vi "BRig_RT_panel_Laser2_v1,13.vi"(7 "input_setValues":bool, 9 "input_dataExp":u16[](array[numeric]), 11 "input_dataLC":u16[](array[numeric])) -> (1 "output_dataExp":u16[](array[numeric]), 3 "output_dataLC":u16[](array[numeric]))   [LabVIEW 2014]
panel:
  in  "LC_Wro_nRew2":u16
  in  "LC_Wro_nRew1":u16
  in  "LC_Rew_nRew2":u16
  in  "LC_Rew_nRew1":u16
  in  "LC_Sel_nRew2":u16
  in  "LC_Sel_nRew1":u16
  in  "LC_Cue2_nRew2":u16
  in  "LC_Cue2_nRew1":u16
  in  "LC_Cue_nRew2":u16
  in  "LC_Cue_nRew1":u16
  in  "LC_ENL2_nRew2":u16
  in  "LC_ENL2_nRew1":u16
  in  "LC_ENL_nRew2":u16
  in  "LC_ENL_nRew1":u16
  in  "LC_Cue2_PostR_Count":u16
  in  "LC_Cue2_PostR_delayOpt":bool
  in  "LC_Cue2_PostR_Probability":u16
  in  "LC_Cue2_PostR_Block":u16(slide) max=2 step=1 scale=0.0..2.0
  in  "LC_Cue2_PostR_OnOff":bool
  in  "LC_Cue2_PostR_Tdelay":u16
  in  "LC_ENL2_PostR_delayOpt":bool
  in  "LC_ENL2_PostR_Count":u16
  in  "LC_ENL2_PostR_Probability":u16 max=100 step=1
  in  "LC_ENL2_PostR_Block":u16(slide) max=2 step=1 scale=0.0..2.0
  in  "LC_ENL2_PostR_OnOff":bool
  in  "LC_ENL2_PostR_Tdelay":u16
  in  "LC_Cue2_PreR_Count":u16
  in  "LC_Cue2_First_Count":u16
  in  "LC_Cue2_PreR_delayOpt":bool
  in  "LC_ENL2_PreR_delayOpt":bool
  in  "LC_ENL2_PreR_Count":u16
  in  "LC_ENL2_First_Count":u16
  in  "LC_Cue2_First_delayOpt":bool
  in  "LC_ENL2_First_delayOpt":bool
  in  "LC_Cue2_PreR_Probability":u16
  in  "LC_Cue2_PreR_Block":u16(slide) max=2 step=1 scale=0.0..2.0
  in  "LC_Cue2_PreR_OnOff":bool
  in  "LC_Cue2_First_Probability":u16
  in  "LC_Cue2_First_Block":u16(slide) max=2 step=1 scale=0.0..2.0
  in  "LC_Cue2_First_OnOff":bool
  in  "LC_ENL2_PreR_Probability":u16 max=100 step=1
  in  "LC_ENL2_PreR_Block":u16(slide) max=2 step=1 scale=0.0..2.0
  in  "LC_ENL2_PreR_OnOff":bool
  in  "LC_ENL2_First_Probability":u16 max=100 step=1
  in  "LC_ENL2_First_Block":u16(slide) max=2 step=1 scale=0.0..2.0
  in  "LC_Cue2_PreR_Tdelay":u16
  in  "LC_ENL2_PreR_Tdelay":u16
  in  "LC_Cue2_First_Tdelay":u16
  in  "LC_ENL2_First_Tdelay":u16
  in  "LC_ENL2_First_OnOff":bool
  out "LaserPulseTrain":cluster{u16[], u16[]}(graph)
  in  "LED_baseline":bool
  in  "Laser_power_step":dbl
  in  "Laser_power_max":dbl
  in  "Laser_power_min":dbl
  in  "Laser_Tshutter":u16=2
  in  "Laser_Freq":u16=10
  in  "Laser_Tpeak":u16=2
  in  "Laser_T":u16
  in  "LC_Sel_PostR_Count":u16
  in  "LC_Sel_PostR_Probability":u16
  in  "LC_Sel_PostR_Block":u16(slide) max=2 step=1 scale=0.0..2.0
  in  "LC_Sel_PostR_OnOff":bool
  in  "LC_Sel_PostR_Tdelay":u16
  in  "LC_Cue_PostR_Count":u16
  in  "LC_Cue_PostR_delayOpt":bool
  in  "LC_Cue_PostR_Probability":u16
  in  "LC_Cue_PostR_Block":u16(slide) max=2 step=1 scale=0.0..2.0
  in  "LC_Cue_PostR_OnOff":bool
  in  "LC_Cue_PostR_Tdelay":u16
  in  "LC_ENL_PostR_delayOpt":bool
  in  "LC_ENL_PostR_Count":u16
  in  "LC_ENL_PostR_Probability":u16 max=100 step=1
  in  "LC_ENL_PostR_Block":u16(slide) max=2 step=1 scale=0.0..2.0
  in  "LC_ENL_PostR_OnOff":bool
  in  "LC_ENL_PostR_Tdelay":u16
  in  "LC_Sel_PreR_Count":u16
  in  "LC_Sel_First_Count":u16
  in  "LC_Sel_PreR_Probability":u16
  in  "LC_Sel_PreR_Block":u16(slide) max=2 step=1 scale=0.0..2.0
  in  "LC_Sel_PreR_OnOff":bool
  in  "LC_Sel_First_Probability":u16
  in  "LC_Sel_First_Block":u16(slide) max=2 step=1 scale=0.0..2.0
  in  "LC_Sel_First_OnOff":bool
  in  "LC_Sel_PreR_Tdelay":u16
  in  "LC_Sel_First_Tdelay":u16
  in  "LC_Cue_PreR_Count":u16
  in  "LC_Cue_First_Count":u16
  in  "LC_Cue_PreR_delayOpt":bool
  in  "LC_ENL_PreR_delayOpt":bool
  in  "LC_ENL_PreR_Count":u16
  in  "LC_ENL_First_Count":u16
  in  "LC_Cue_First_delayOpt":bool
  in  "LC_ENL_First_delayOpt":bool
  in  "LC_Wrong_Probability":u16
  in  "LC_Wrong_Trial":u16(slide) max=4 step=1 scale=0.0..4.0
  in  "LC_Wrong_Block":u16(slide) max=2 step=1 scale=0.0..2.0
  in  "LC_Wrong_OnOff":bool
  in  "LC_Reward_Probability":u16
  in  "LC_Reward_Trial":u16(slide) max=3 step=1 scale=0.0..3.0
  in  "LC_Reward_Block":u16(slide) max=2 step=1 scale=0.0..2.0
  in  "LC_Reward_OnOff":bool
  in  "LC_Cue_PreR_Probability":u16
  in  "LC_Cue_PreR_Block":u16(slide) max=2 step=1 scale=0.0..2.0
  in  "LC_Cue_PreR_OnOff":bool
  in  "LC_Cue_First_Probability":u16
  in  "LC_Cue_First_Block":u16(slide) max=2 step=1 scale=0.0..2.0
  in  "LC_Cue_First_OnOff":bool
  in  "LC_ENL_PreR_Probability":u16 max=100 step=1
  in  "LC_ENL_PreR_Block":u16(slide) max=2 step=1 scale=0.0..2.0
  in  "LC_ENL_PreR_OnOff":bool
  in  "LC_ENL_First_Probability":u16 max=100 step=1
  in  "LC_ENL_First_Block":u16(slide) max=2 step=1 scale=0.0..2.0
  in  "LC_Wrong_Tdelay":u16
  in  "LC_Cue_PreR_Tdelay":u16
  in  "LC_ENL_PreR_Tdelay":u16
  in  "LC_Reward_Tdelay":u16
  in  "LC_Cue_First_Tdelay":u16
  in  "LC_ENL_First_Tdelay":u16
  in  "LC_ENL_First_OnOff":bool
  # "Laser2 Control\n                               On/Off      Block        Probability [%]   Delay [ms]                              Count"
  # "On/Off      Block        Probability [%]   Delay [ms]                              Count"
  # "Enforced\nNonLick"
  # "Enforced\nNonLick\n     2"
  # "from end"
  # "from end"
  # "First\nTrial"
  # "First\nTrial"
  # "from start"
  # "from start"
  # "from end"
  # "from end"
  # "PreReward\nTrials"
  # "PreReward\nTrials"
  # "from start"
  # "from start"
  # "from end"
  # "from end"
  # "PostReward\nTrials"
  # "PostReward\nTrials"
  # "from start"
  # "from start"
  # "PostReward Option - Trigger after [X1] or [X2] reward\n                                        (0 = ignore this option)"
  # "PostReward Option - Trigger after [X1] or [X2] reward\n                                        (0 = ignore this option)"
  # "Cue"
  # "Cue\n  2"
  # "from end"
  # "from end"
  # "First\nTrial"
  # "First\nTrial"
  # "from start"
  # "from start"
  # "from end"
  # "from end"
  # "PreReward\nTrials"
  # "PreReward\nTrials"
  # "from start"
  # "from start"
  # "from end"
  # "from end"
  # "PostReward\nTrials"
  # "PostReward\nTrials"
  # "from start"
  # "from start"
  # "PostReward Option - Trigger after [X1] or [X2] reward\n                                        (0 = ignore this option)"
  # "PostReward Option - Trigger after [X1] or [X2] reward\n                                        (0 = ignore this option)"
  # "Selection"
  # "from start"
  # "First\nTrial"
  # "from start"
  # "PreReward\nTrials"
  # "from start"
  # "PostReward\nTrials"
  # "PostReward Option - Trigger after [X1] or [X2] reward\n                                        (0 = ignore this option)"
  # "Laser2 Parameters"
  # "Laser2 Response\n           On/Off      Block           Trial     Probability %  Delay [ms]"
  # "Frequency\n[Hz]"
  # "Selection\nReward"
  # "Timing [ms]\n Duration     Peak Width   Shutter"
  # "Trigger after [X1] or [X2] reward\n(0 = ignore this option)"
  # "Laser Power [V]\nMin          Max              Step"
  # "Selection\nWrong"
  # "Trigger after [X1] or [X2] reward\n(0 = ignore this option)"
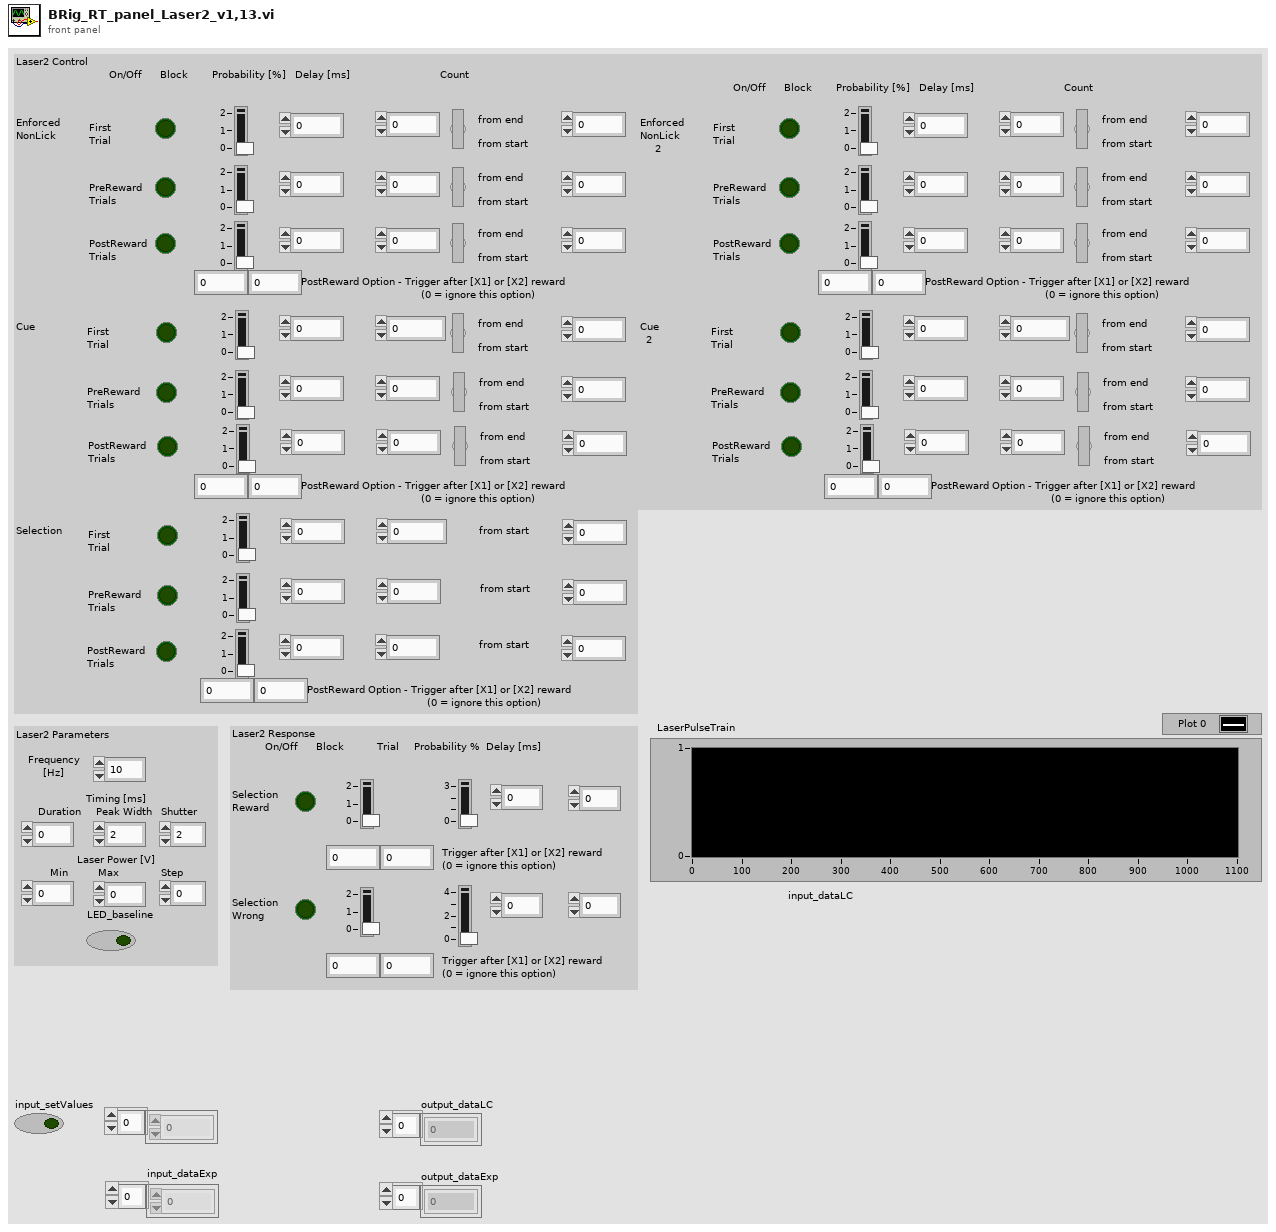
[diagram p1: front panel]
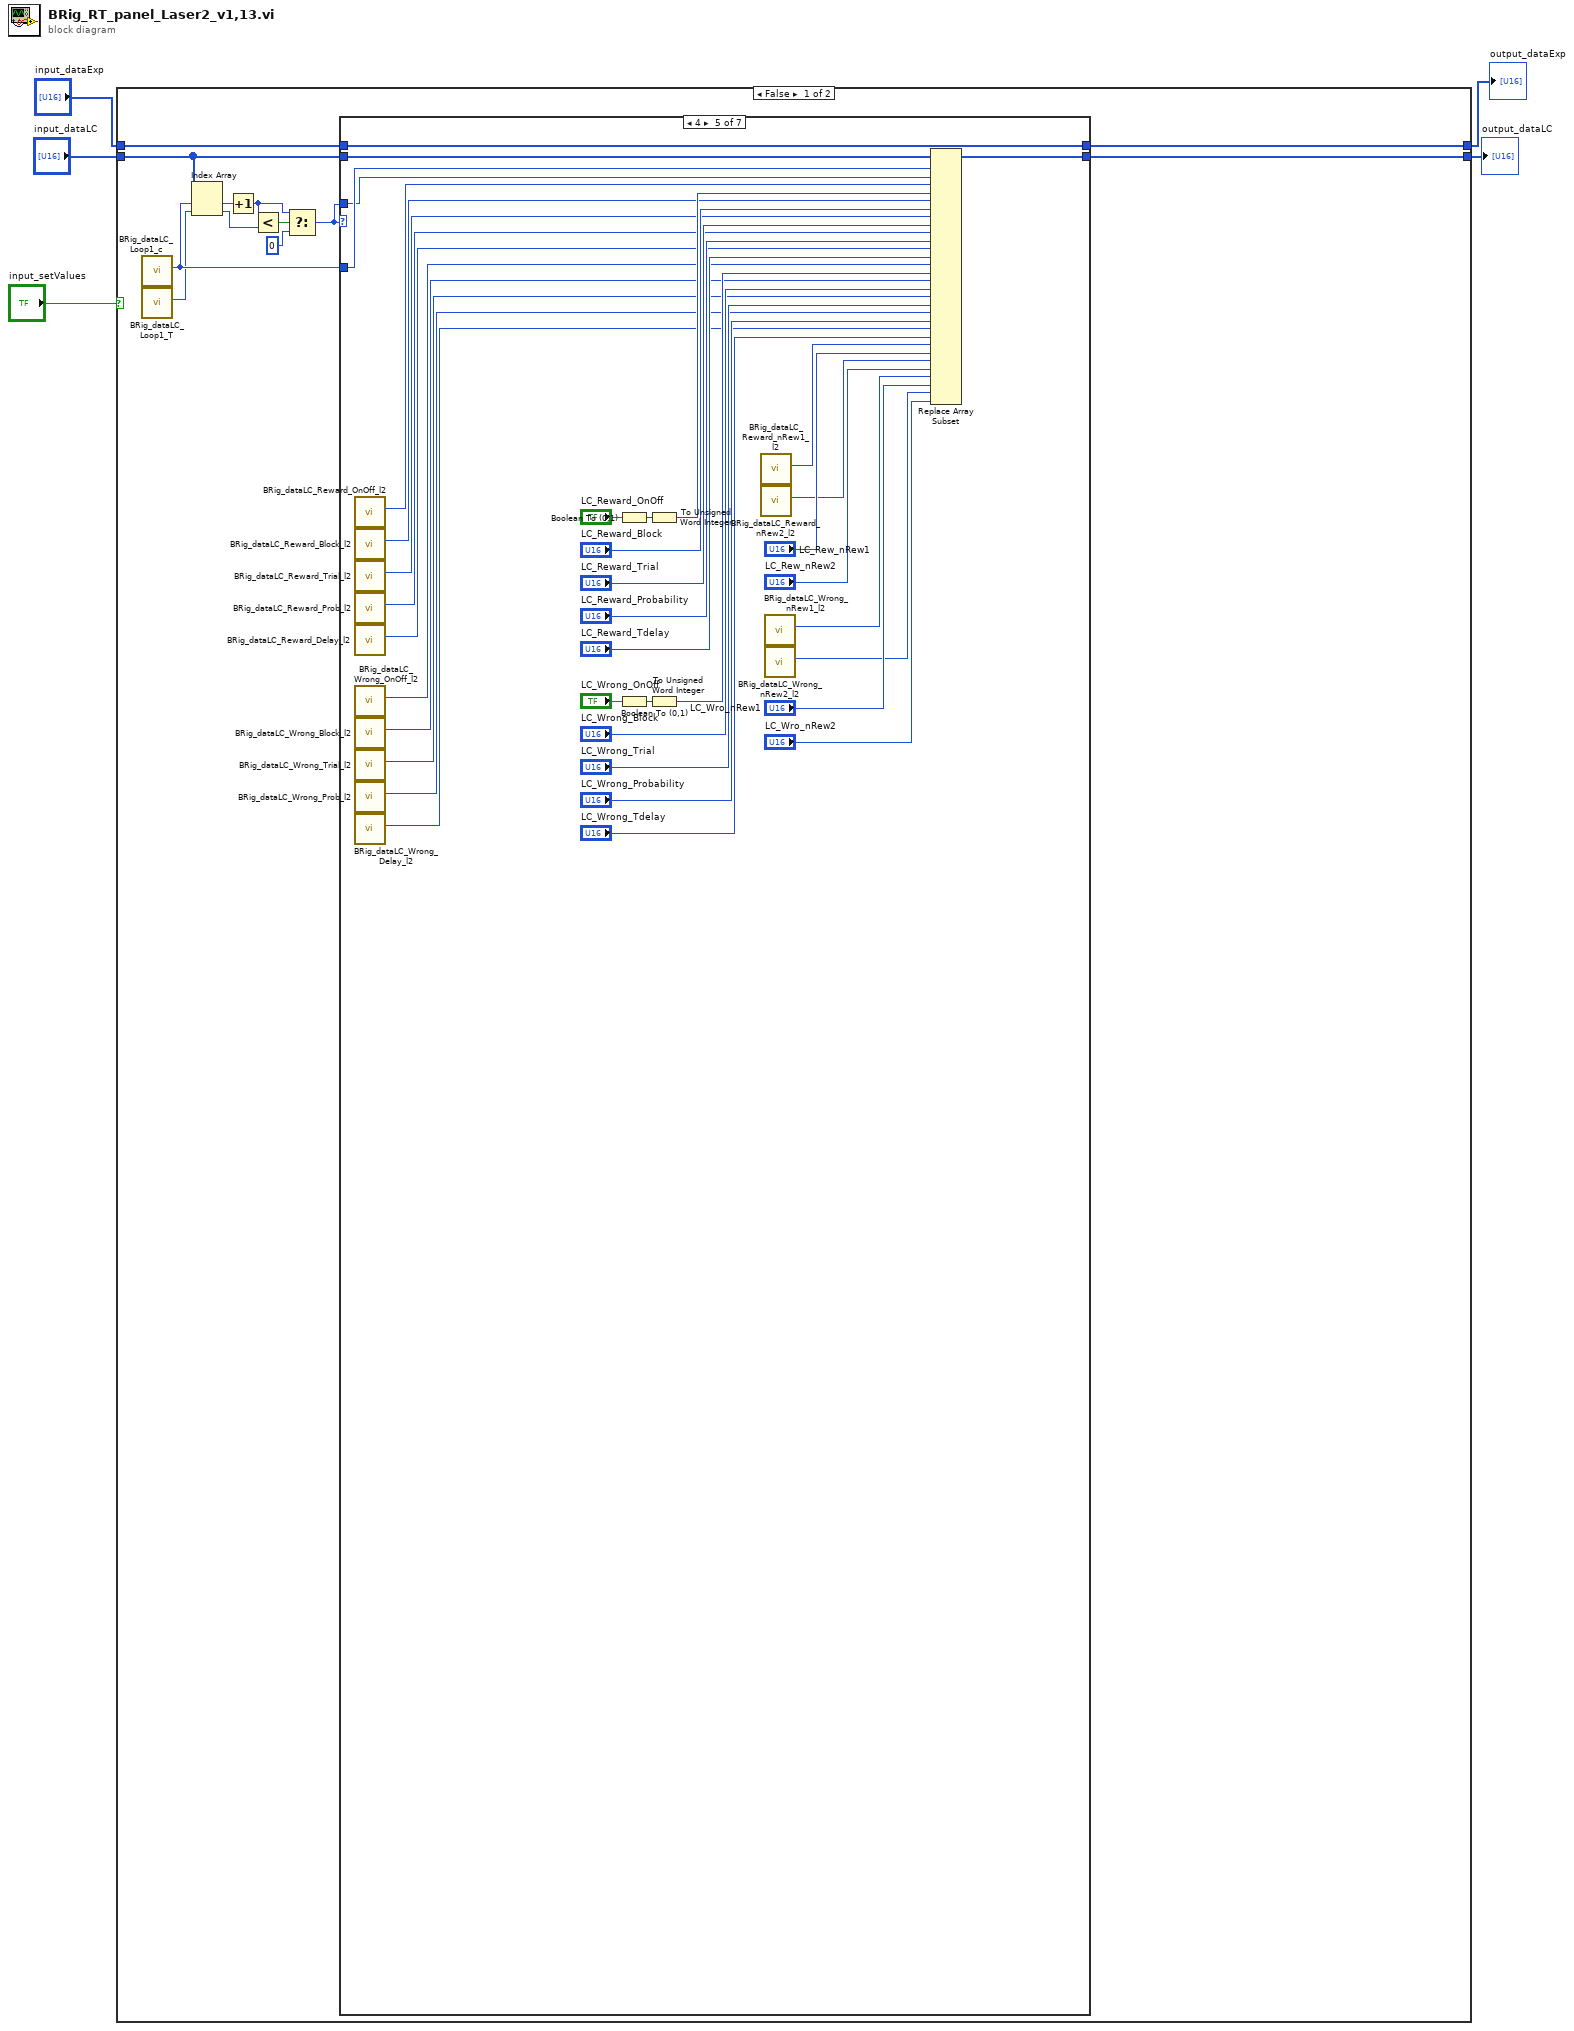
[diagram p0: block diagram]
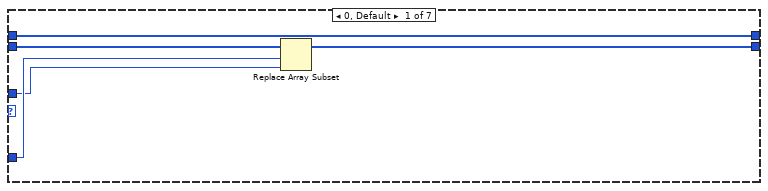
[diagram p2: hidden frame]
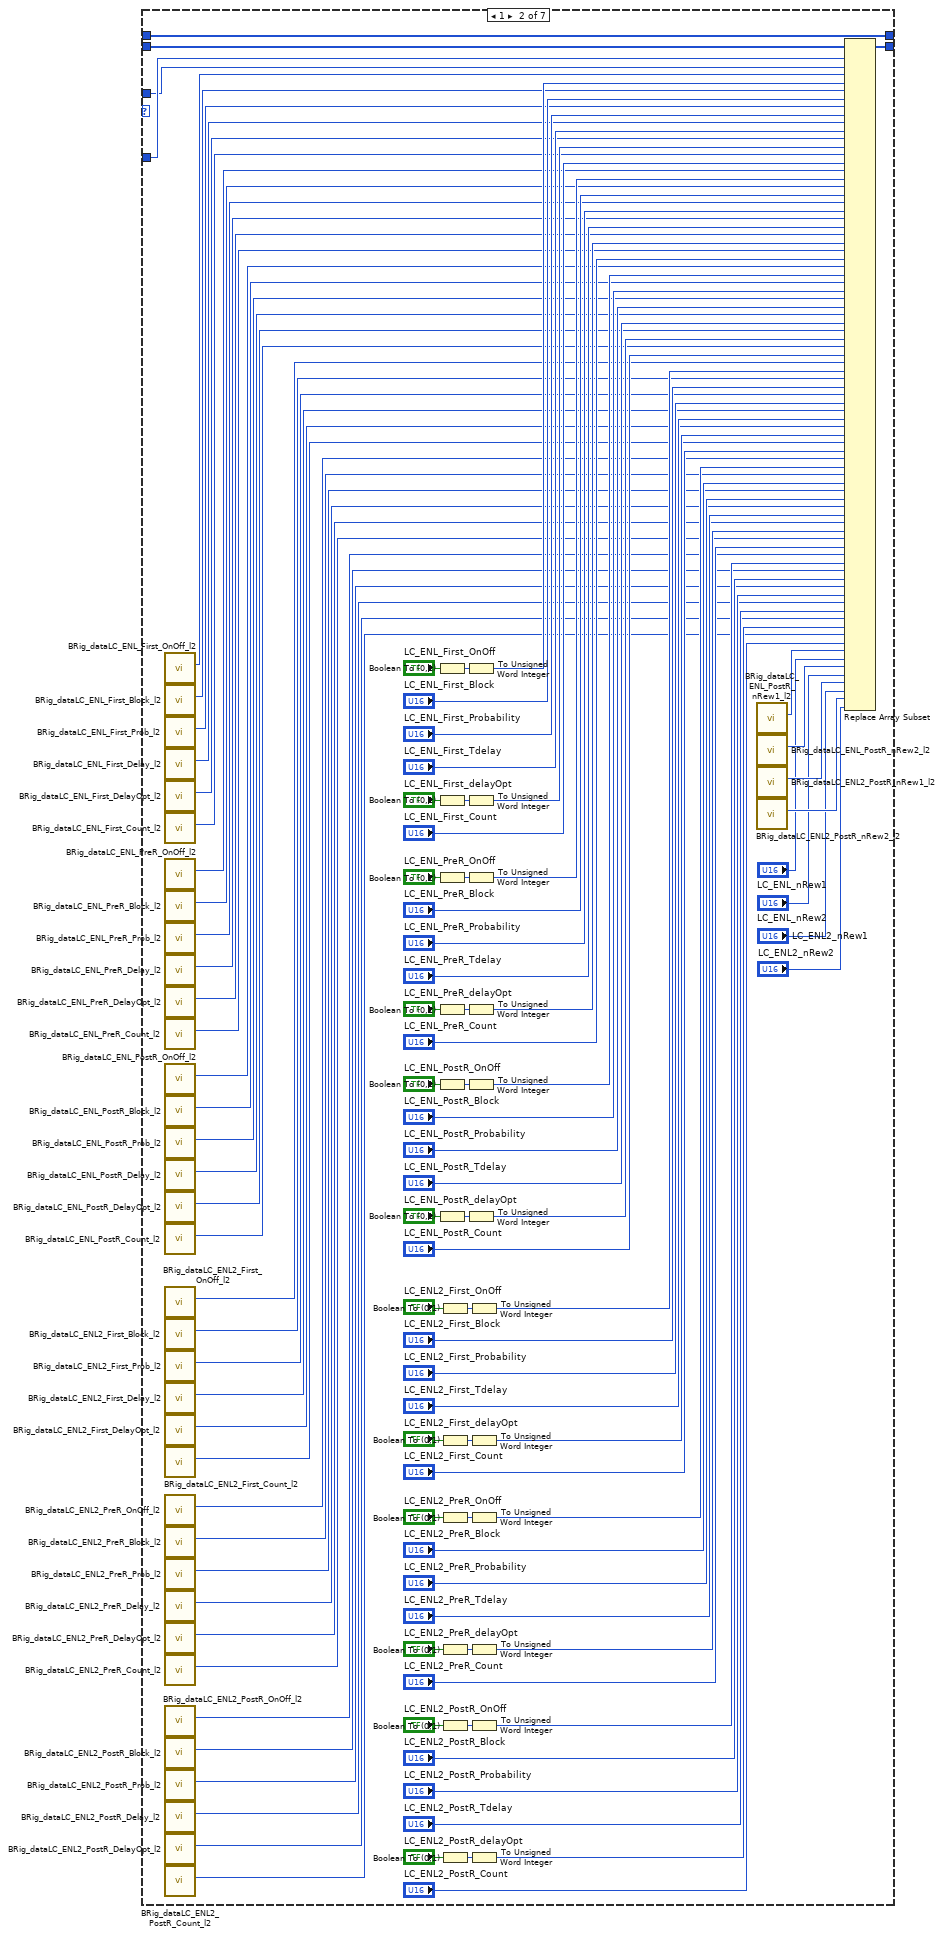
[diagram p3: hidden frame]
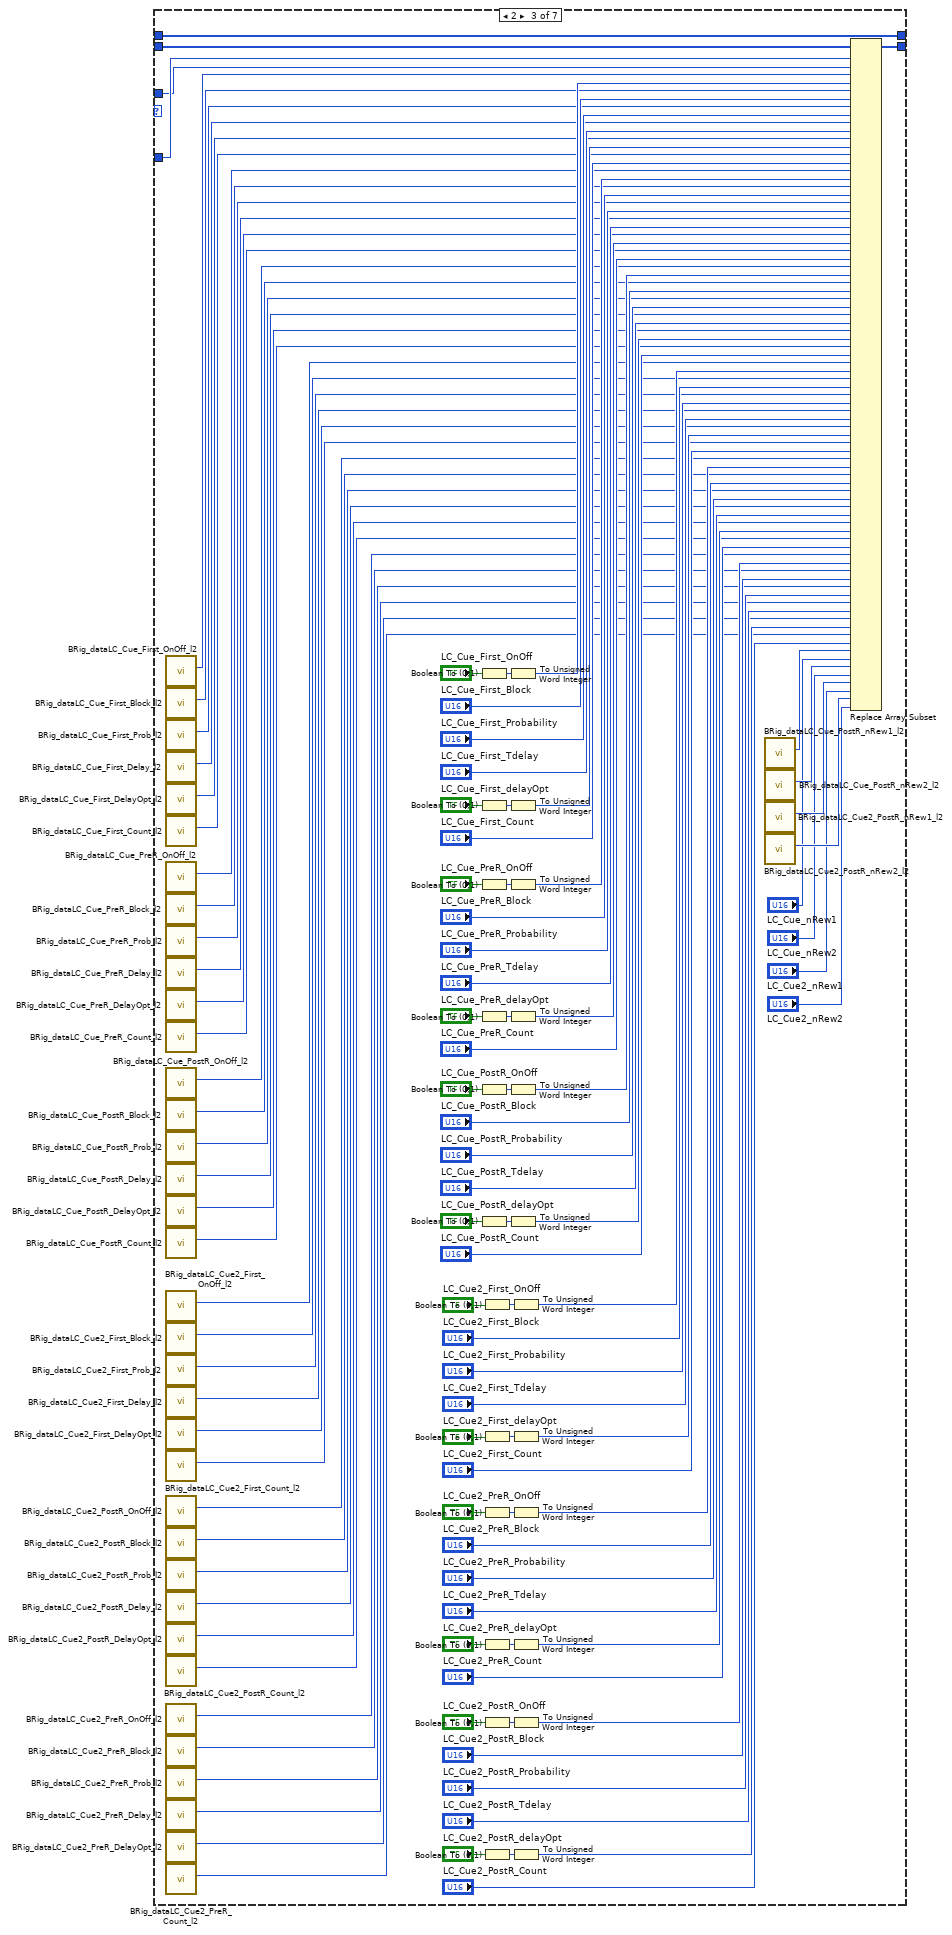
[diagram p4: hidden frame]
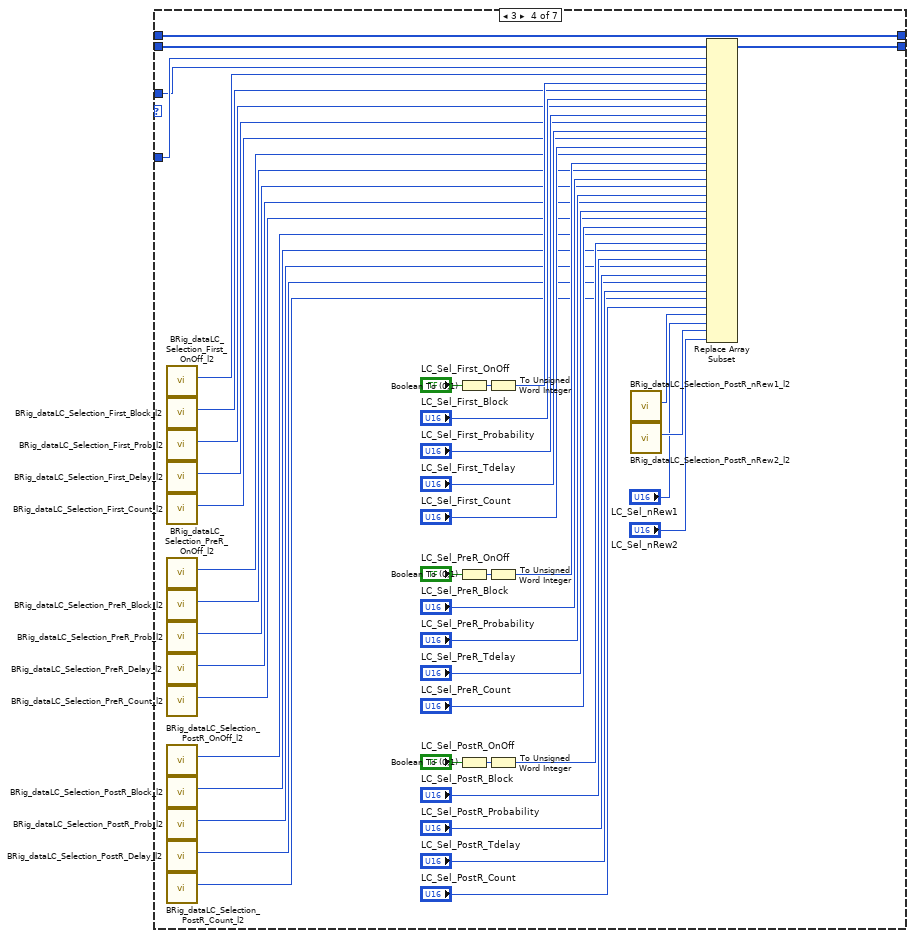
[diagram p5: hidden frame]
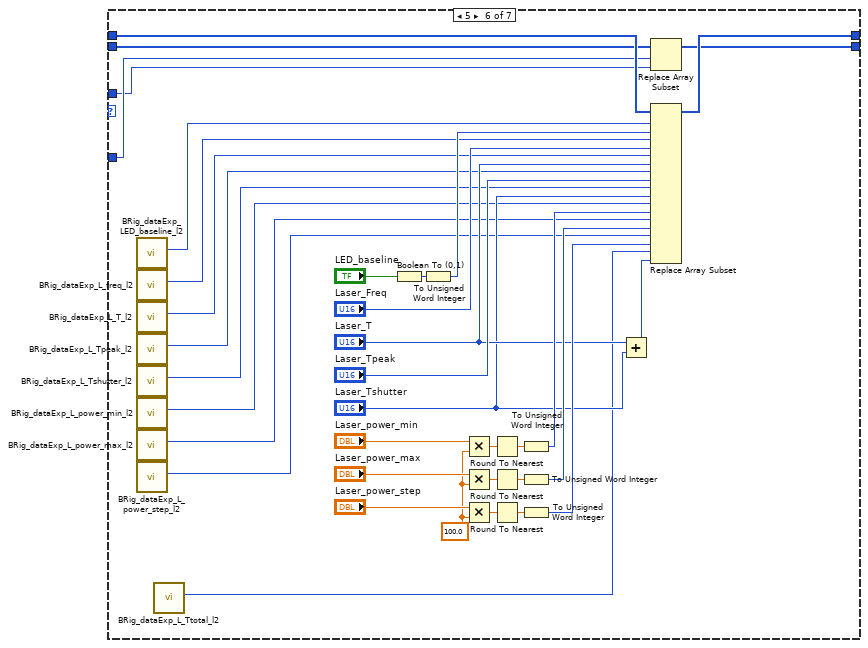
[diagram p6: hidden frame]
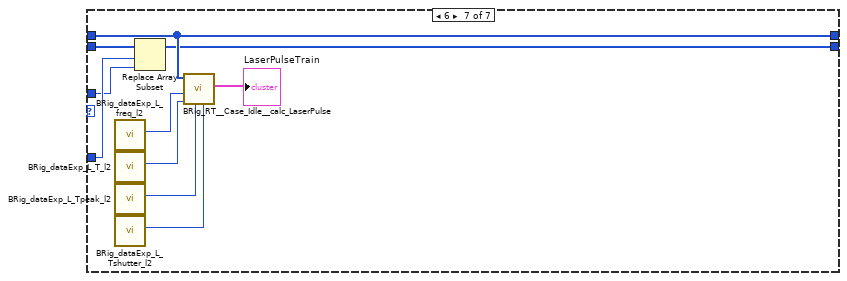
[diagram p7: hidden frame]
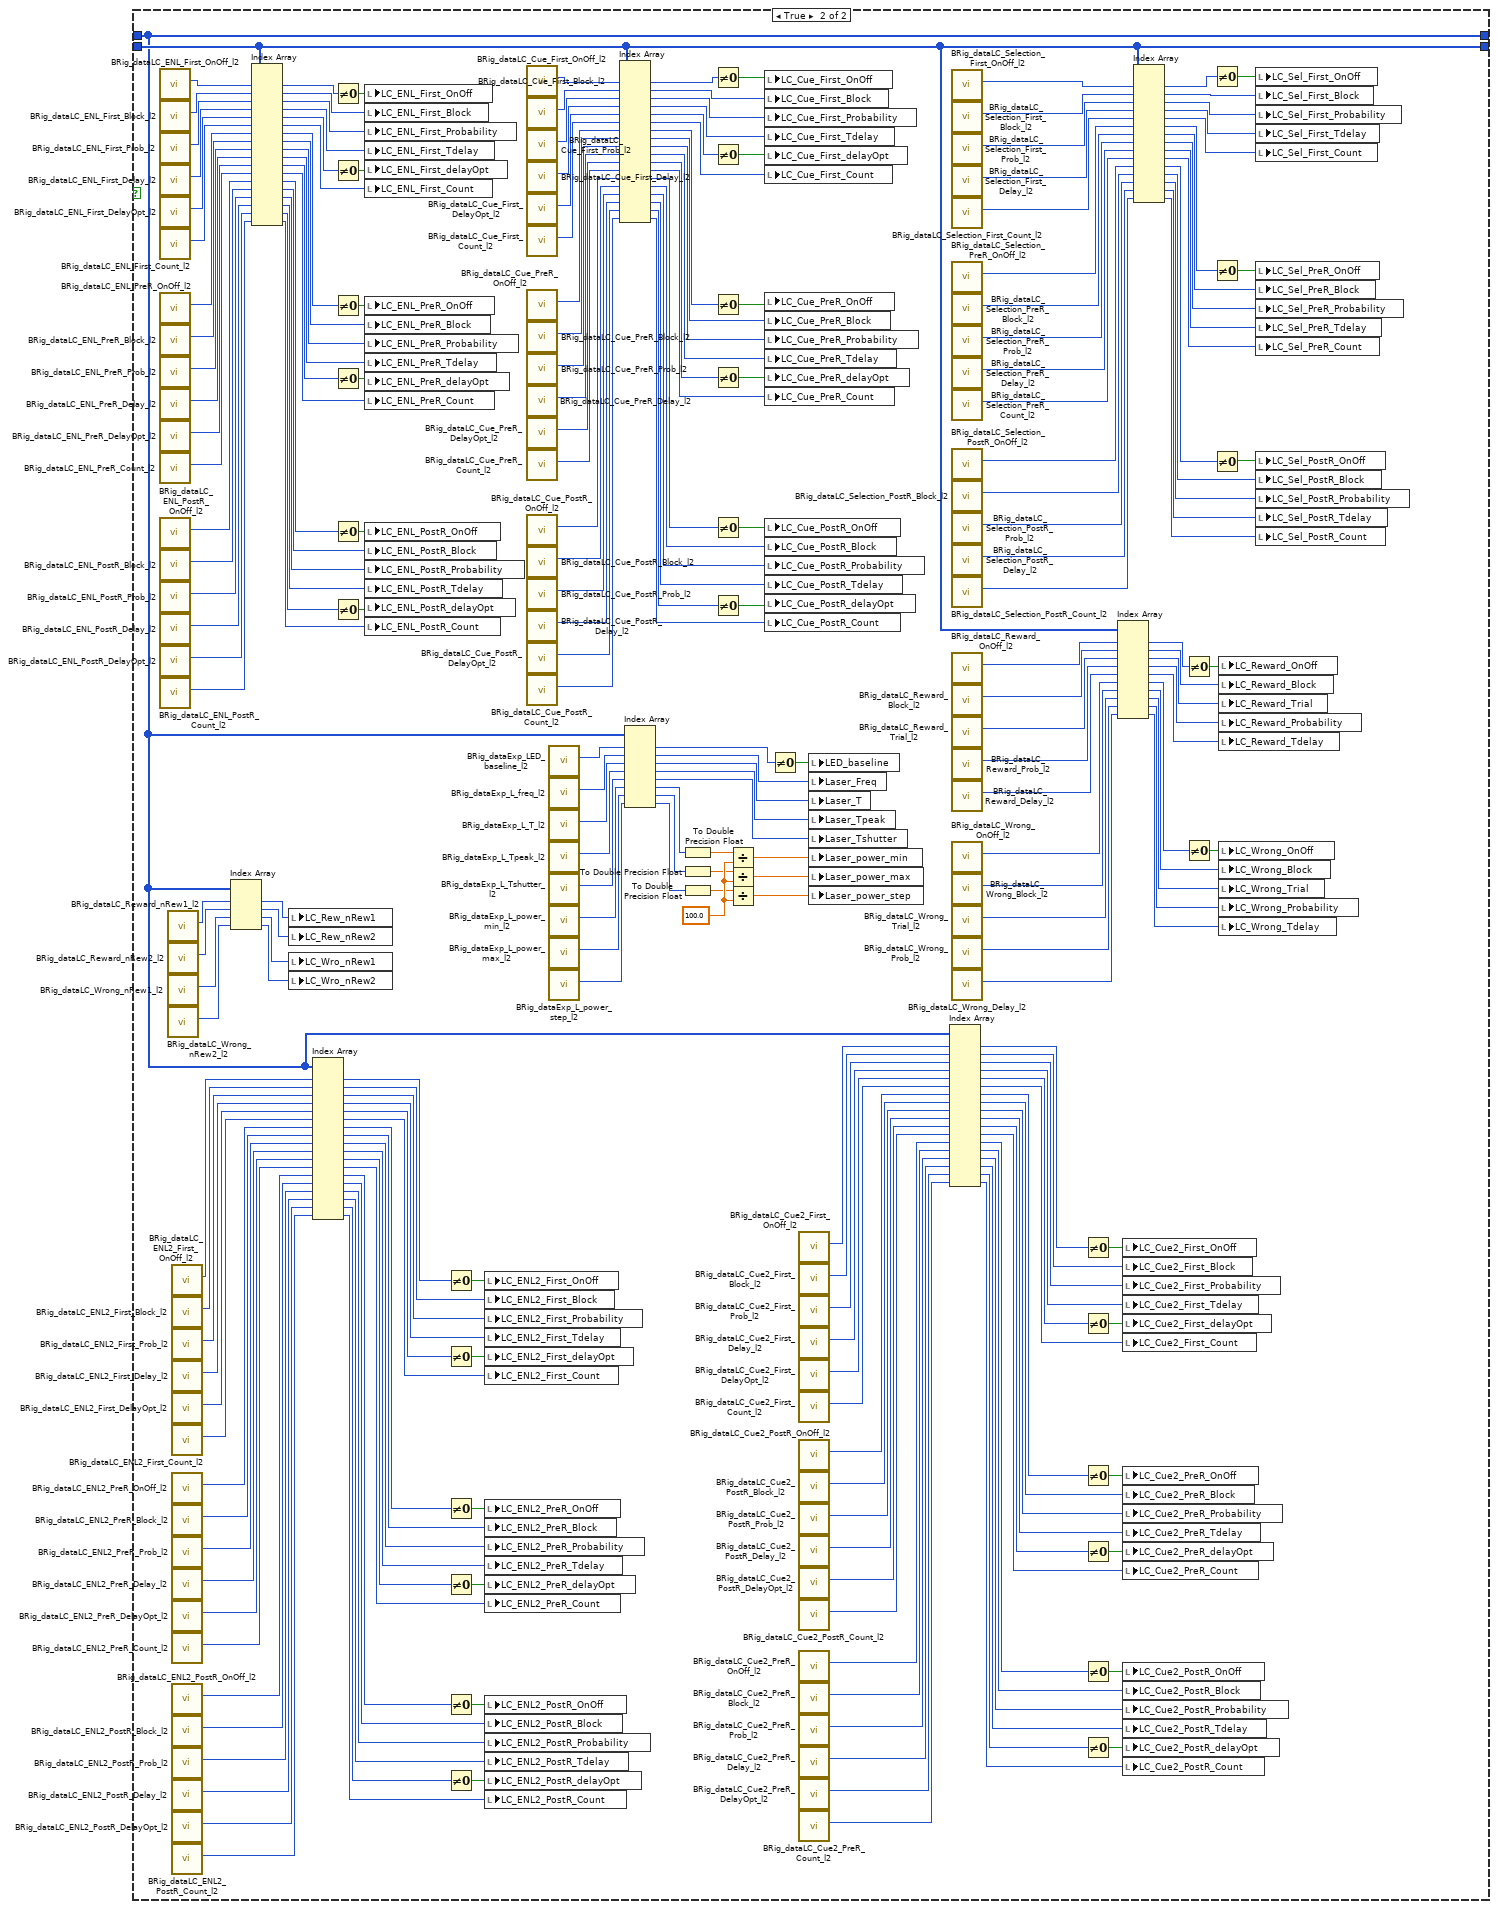
[diagram p8: hidden frame]
diagram:
  n1 = case shown="False" "input_setValues" {
    tunnel: "input_dataLC" -> [w17 w547]
    tunnel: [w11 w547] -> w4
    tunnel: "input_dataExp" -> [w7 w377]
    tunnel: [w6 w377] -> w1
    frame False {
      n2 = call "BRig_dataLC_Loop1_c.vi"() -> ("output_Loop1_c"=w10:i32)  [unwired: 11 in]
      n3 = call "BRig_dataLC_Loop1_T.vi"() -> ("output_Loop1_T"=w9:i32)  [unwired: 11 in]
      n4 = Index Array(array=w17, index #1=w10, index #2=w9) -> (element #1=w16:u16, element #2=w15:u16)
      n5 = Increment(x=w16) -> (x+1=w12:u16)
      n6 = Less?(x=w12, y=w15) -> (x < y?=w14:bool)
      n7 = Select(t=w12, s=w14, f=u16 0) -> (s? t:f=w8:u16)
      n8 = case shown="4" w8 {
        tunnel: w17 -> [w22 w131 w240 w285 w322 w335 w366]
        tunnel: w10 -> [w20 w99 w208 w262 w306 w333 w364]
        tunnel: w8 -> [w19 w98 w207 w261 w305 w332 w363]
        tunnel: [w21 w130 w239 w284 w321 w334 w365] -> w11
        tunnel: w7 -> [w18 w97 w206 w260 w304 w337 w368]
        tunnel: [w18 w97 w206 w260 w304 w336 w368] -> w6
        frame 0, Default {
          n9 = Replace Array Subset(array=w22, new element=w19, index=w20) -> (w21:u16[])
        }
        frame 1 {
          n10 = call "BRig_dataLC_ENL_First_OnOff_l2.vi"() -> ("output_ENL_First_OnOff_l2"=w49:i32)  [unwired: 11 in]
          n11 = call "BRig_dataLC_ENL_First_Block_l2.vi"() -> ("output_ENL_First_Block_l2"=w50:i32)  [unwired: 11 in]
          n12 = call "BRig_dataLC_ENL_First_Prob_l2.vi"() -> ("output_ENL_First_Prob_l2"=w51:i32)  [unwired: 11 in]
          n13 = call "BRig_dataLC_ENL_First_Delay_l2.vi"() -> ("output_ENL_First_Delay_l2"=w52:i32)  [unwired: 11 in]
          n14 = call "BRig_dataLC_ENL_First_DelayOpt_l2.vi"() -> ("output_ENL_First_DelayOpt_l2"=w53:i32)  [unwired: 11 in]
          n15 = call "BRig_dataLC_ENL_First_Count_l2.vi"() -> ("output_ENL_First_Count_l2"=w54:i32)  [unwired: 11 in]
          n16 = call "BRig_dataLC_ENL_PreR_OnOff_l2.vi"() -> ("output_ENL_PreR_OnOff_l2"=w55:i32)  [unwired: 11 in]
          n17 = call "BRig_dataLC_ENL_PreR_Block_l2.vi"() -> ("output_ENL_PreR_Block_l2"=w56:i32)  [unwired: 11 in]
          n18 = call "BRig_dataLC_ENL_PreR_Prob_l2.vi"() -> ("output_ENL_PreR_Prob_l2"=w57:i32)  [unwired: 11 in]
          n19 = call "BRig_dataLC_ENL_PreR_Delay_l2.vi"() -> ("output_ENL_PreR_Delay_l2"=w58:i32)  [unwired: 11 in]
          n20 = call "BRig_dataLC_ENL_PreR_DelayOpt_l2.vi"() -> ("output_ENL_PreR_DelayOpt_l2"=w59:i32)  [unwired: 11 in]
          n21 = call "BRig_dataLC_ENL_PreR_Count_l2.vi"() -> ("output_ENL_PreR_Count_l2"=w60:i32)  [unwired: 11 in]
          n22 = call "BRig_dataLC_ENL_PostR_OnOff_l2.vi"() -> ("output_ENL_PostR_OnOff_l2"=w61:i32)  [unwired: 11 in]
          n23 = call "BRig_dataLC_ENL_PostR_Block_l2.vi"() -> ("output_ENL_PostR_Block_l2"=w62:i32)  [unwired: 11 in]
          n24 = call "BRig_dataLC_ENL_PostR_Prob_l2.vi"() -> ("output_ENL_PostR_Prob_l2"=w63:i32)  [unwired: 11 in]
          n25 = call "BRig_dataLC_ENL_PostR_Delay_l2.vi"() -> ("output_ENL_PostR_Delay_l2"=w64:i32)  [unwired: 11 in]
          n26 = call "BRig_dataLC_ENL_PostR_DelayOpt_l2.vi"() -> ("output_ENL_PostR_DelayOpt_l2"=w65:i32)  [unwired: 11 in]
          n27 = call "BRig_dataLC_ENL_PostR_Count_l2.vi"() -> ("output_ENL_PostR_Count_l2"=w66:i32)  [unwired: 11 in]
          n28 = call "BRig_dataLC_ENL2_First_OnOff_l2.vi"() -> ("output_ENL2_First_OnOff_l2"=w48:i32)  [unwired: 11 in]
          n29 = call "BRig_dataLC_ENL2_First_Block_l2.vi"() -> ("output_ENL2_First_Block_l2"=w47:i32)  [unwired: 11 in]
          n30 = call "BRig_dataLC_ENL2_First_Prob_l2.vi"() -> ("output_ENL2_First_Prob_l2"=w46:i32)  [unwired: 11 in]
          n31 = call "BRig_dataLC_ENL2_First_Delay_l2.vi"() -> ("output_ENL2_First_Delay_l2"=w45:i32)  [unwired: 11 in]
          n32 = call "BRig_dataLC_ENL2_First_DelayOpt_l2.vi"() -> ("output_ENL2_First_DelayOpt_l2"=w44:i32)  [unwired: 11 in]
          n33 = call "BRig_dataLC_ENL2_First_Count_l2.vi"() -> ("output_ENL2_First_Count_l2"=w43:i32)  [unwired: 11 in]
          n34 = call "BRig_dataLC_ENL2_PreR_OnOff_l2.vi"() -> ("output_ENL2_PreR_OnOff_l2"=w42:i32)  [unwired: 11 in]
          n35 = call "BRig_dataLC_ENL2_PreR_Block_l2.vi"() -> ("output_ENL2_PreR_Block_l2"=w41:i32)  [unwired: 11 in]
          n36 = call "BRig_dataLC_ENL2_PreR_Prob_l2.vi"() -> ("output_ENL2_PreR_Prob_l2"=w40:i32)  [unwired: 11 in]
          n37 = call "BRig_dataLC_ENL2_PreR_Delay_l2.vi"() -> ("output_ENL2_PreR_Delay_l2"=w39:i32)  [unwired: 11 in]
          n38 = call "BRig_dataLC_ENL2_PreR_DelayOpt_l2.vi"() -> ("output_ENL2_PreR_DelayOpt_l2"=w38:i32)  [unwired: 11 in]
          n39 = call "BRig_dataLC_ENL2_PreR_Count_l2.vi"() -> ("output_ENL2_PreR_Count_l2"=w37:i32)  [unwired: 11 in]
          n40 = call "BRig_dataLC_ENL2_PostR_OnOff_l2.vi"() -> ("output_ENL2_PostR_OnOff_l2"=w36:i32)  [unwired: 11 in]
          n41 = call "BRig_dataLC_ENL2_PostR_Block_l2.vi"() -> ("output_ENL2_PostR_Block_l2"=w35:i32)  [unwired: 11 in]
          n42 = call "BRig_dataLC_ENL2_PostR_Prob_l2.vi"() -> ("output_ENL2_PostR_Prob_l2"=w34:i32)  [unwired: 11 in]
          n43 = call "BRig_dataLC_ENL2_PostR_Delay_l2.vi"() -> ("output_ENL2_PostR_Delay_l2"=w33:i32)  [unwired: 11 in]
          n44 = call "BRig_dataLC_ENL2_PostR_DelayOpt_l2.vi"() -> ("output_ENL2_PostR_DelayOpt_l2"=w32:i32)  [unwired: 11 in]
          n45 = call "BRig_dataLC_ENL2_PostR_Count_l2.vi"() -> ("output_ENL2_PostR_Count_l2"=w31:i32)  [unwired: 11 in]
          n46 = Boolean To (0,1)(Boolean="LC_ENL_First_OnOff") -> (0, 1=w128:i16)
          n47 = Boolean To (0,1)(Boolean="LC_ENL_First_delayOpt") -> (0, 1=w127:i16)
          n48 = Boolean To (0,1)(Boolean="LC_ENL_PreR_OnOff") -> (0, 1=w125:i16)
          n49 = Boolean To (0,1)(Boolean="LC_ENL_PreR_delayOpt") -> (0, 1=w123:i16)
          n50 = Boolean To (0,1)(Boolean="LC_ENL_PostR_OnOff") -> (0, 1=w121:i16)
          n51 = Boolean To (0,1)(Boolean="LC_ENL_PostR_delayOpt") -> (0, 1=w119:i16)
          n52 = Boolean To (0,1)(Boolean="LC_ENL2_First_OnOff") -> (0, 1=w87:i16)
          n53 = Boolean To (0,1)(Boolean="LC_ENL2_First_delayOpt") -> (0, 1=w86:i16)
          n54 = Boolean To (0,1)(Boolean="LC_ENL2_PreR_OnOff") -> (0, 1=w85:i16)
          n55 = Boolean To (0,1)(Boolean="LC_ENL2_PreR_delayOpt") -> (0, 1=w83:i16)
          n56 = Boolean To (0,1)(Boolean="LC_ENL2_PostR_OnOff") -> (0, 1=w75:i16)
          n57 = Boolean To (0,1)(Boolean="LC_ENL2_PostR_delayOpt") -> (0, 1=w73:i16)
          n58 = To Unsigned Word Integer(number=w128) -> (unsigned 16bit integer=w117:u16)
          n59 = To Unsigned Word Integer(number=w127) -> (unsigned 16bit integer=w113:u16)
          n60 = To Unsigned Word Integer(number=w125) -> (unsigned 16bit integer=w111:u16)
          n61 = To Unsigned Word Integer(number=w123) -> (unsigned 16bit integer=w107:u16)
          n62 = To Unsigned Word Integer(number=w121) -> (unsigned 16bit integer=w105:u16)
          n63 = To Unsigned Word Integer(number=w119) -> (unsigned 16bit integer=w101:u16)
          n64 = To Unsigned Word Integer(number=w87) -> (unsigned 16bit integer=w94:u16)
          n65 = To Unsigned Word Integer(number=w86) -> (unsigned 16bit integer=w90:u16)
          n66 = To Unsigned Word Integer(number=w85) -> (unsigned 16bit integer=w88:u16)
          n67 = To Unsigned Word Integer(number=w83) -> (unsigned 16bit integer=w78:u16)
          n68 = To Unsigned Word Integer(number=w75) -> (unsigned 16bit integer=w76:u16)
          n69 = To Unsigned Word Integer(number=w73) -> (unsigned 16bit integer=w68:u16)
          n70 = call "BRig_dataLC_ENL_PostR_nRew1_l2.vi"() -> ("output_ENL_PostR_nRew1_l2"=w30:i32)  [unwired: 11 in]
          n71 = call "BRig_dataLC_ENL_PostR_nRew2_l2.vi"() -> ("output_ENL_PostR_nRew2_l2"=w29:i32)  [unwired: 11 in]
          n72 = call "BRig_dataLC_ENL2_PostR_nRew1_l2.vi"() -> ("output_ENL2_PostR_nRew1_l2"=w28:i32)  [unwired: 11 in]
          n73 = call "BRig_dataLC_ENL2_PostR_nRew2_l2.vi"() -> ("output_ENL2_PostR_nRew2_l2"=w27:i32)  [unwired: 11 in]
          n74 = Replace Array Subset(array=w131, new element #1=w98, index #1=w99, new element #2=w117, index #2=w49, new element #3="LC_ENL_First_Block", index #3=w50, new element #4="LC_ENL_First_Probability", index #4=w51, new element #5="LC_ENL_First_Tdelay", index #5=w52, new element #6=w113, index #6=w53, new element #7="LC_ENL_First_Count", index #7=w54, new element #8=w111, index #8=w55, new element #9="LC_ENL_PreR_Block", index #9=w56, new element #10="LC_ENL_PreR_Probability", index #10=w57, new element #11="LC_ENL_PreR_Tdelay", index #11=w58, new element #12=w107, index #12=w59, new element #13="LC_ENL_PreR_Count", index #13=w60, new element #14=w105, index #14=w61, new element #15="LC_ENL_PostR_Block", index #15=w62, new element #16="LC_ENL_PostR_Probability", index #16=w63, new element #17="LC_ENL_PostR_Tdelay", index #17=w64, new element #18=w101, index #18=w65, new element #19="LC_ENL_PostR_Count", index #19=w66, new element #20=w94, index #20=w48, new element #21="LC_ENL2_First_Block", index #21=w47, new element #22="LC_ENL2_First_Probability", index #22=w46, new element #23="LC_ENL2_First_Tdelay", index #23=w45, new element #24=w90, index #24=w44, new element #25="LC_ENL2_First_Count", index #25=w43, new element #26=w88, index #26=w42, new element #27="LC_ENL2_PreR_Block", index #27=w41, new element #28="LC_ENL2_PreR_Probability", index #28=w40, new element #29="LC_ENL2_PreR_Tdelay", index #29=w39, new element #30=w78, index #30=w38, new element #31="LC_ENL2_PreR_Count", index #31=w37, new element #32=w76, index #32=w36, new element #33="LC_ENL2_PostR_Block", index #33=w35, new element #34="LC_ENL2_PostR_Probability", index #34=w34, new element #35="LC_ENL2_PostR_Tdelay", index #35=w33, new element #36=w68, index #36=w32, new element #37="LC_ENL2_PostR_Count", index #37=w31, new element #38="LC_ENL_nRew1", index #38=w30, new element #39="LC_ENL_nRew2", index #39=w29, new element #40="LC_ENL2_nRew1", index #40=w28, new element #41="LC_ENL2_nRew2", index #41=w27) -> (w130:u16[])
        }
        frame 2 {
          n75 = call "BRig_dataLC_Cue_First_OnOff_l2.vi"() -> ("output_Cue_First_OnOff_l2"=w158:i32)  [unwired: 11 in]
          n76 = call "BRig_dataLC_Cue_First_Block_l2.vi"() -> ("output_Cue_First_Block_l2"=w159:i32)  [unwired: 11 in]
          n77 = call "BRig_dataLC_Cue_First_Prob_l2.vi"() -> ("output_Cue_First_Prob_l2"=w160:i32)  [unwired: 11 in]
          n78 = call "BRig_dataLC_Cue_First_Delay_l2.vi"() -> ("output_Cue_First_Delay_l2"=w161:i32)  [unwired: 11 in]
          n79 = call "BRig_dataLC_Cue_First_DelayOpt_l2.vi"() -> ("output_Cue_First_DelayOpt_l2"=w162:i32)  [unwired: 11 in]
          n80 = call "BRig_dataLC_Cue_First_Count_l2.vi"() -> ("output_Cue_First_Count_l2"=w163:i32)  [unwired: 11 in]
          n81 = call "BRig_dataLC_Cue_PreR_OnOff_l2.vi"() -> ("output_Cue_PreR_OnOff_l2"=w164:i32)  [unwired: 11 in]
          n82 = call "BRig_dataLC_Cue_PreR_Block_l2.vi"() -> ("output_Cue_PreR_Block_l2"=w165:i32)  [unwired: 11 in]
          n83 = call "BRig_dataLC_Cue_PreR_Prob_l2.vi"() -> ("output_Cue_PreR_Prob_l2"=w166:i32)  [unwired: 11 in]
          n84 = call "BRig_dataLC_Cue_PreR_Delay_l2.vi"() -> ("output_Cue_PreR_Delay_l2"=w167:i32)  [unwired: 11 in]
          n85 = call "BRig_dataLC_Cue_PreR_DelayOpt_l2.vi"() -> ("output_Cue_PreR_DelayOpt_l2"=w168:i32)  [unwired: 11 in]
          n86 = call "BRig_dataLC_Cue_PreR_Count_l2.vi"() -> ("output_Cue_PreR_Count_l2"=w169:i32)  [unwired: 11 in]
          n87 = call "BRig_dataLC_Cue_PostR_OnOff_l2.vi"() -> ("output_Cue_PostR_OnOff_l2"=w170:i32)  [unwired: 11 in]
          n88 = call "BRig_dataLC_Cue_PostR_Block_l2.vi"() -> ("output_Cue_PostR_Block_l2"=w171:i32)  [unwired: 11 in]
          n89 = call "BRig_dataLC_Cue_PostR_Prob_l2.vi"() -> ("output_Cue_PostR_Prob_l2"=w172:i32)  [unwired: 11 in]
          n90 = call "BRig_dataLC_Cue_PostR_Delay_l2.vi"() -> ("output_Cue_PostR_Delay_l2"=w173:i32)  [unwired: 11 in]
          n91 = call "BRig_dataLC_Cue_PostR_DelayOpt_l2.vi"() -> ("output_Cue_PostR_DelayOpt_l2"=w174:i32)  [unwired: 11 in]
          n92 = call "BRig_dataLC_Cue_PostR_Count_l2.vi"() -> ("output_Cue_PostR_Count_l2"=w175:i32)  [unwired: 11 in]
          n93 = call "BRig_dataLC_Cue2_First_OnOff_l2.vi"() -> ("output_Cue2_First_OnOff_l2"=w157:i32)  [unwired: 11 in]
          n94 = call "BRig_dataLC_Cue2_First_Block_l2.vi"() -> ("output_Cue2_First_Block_l2"=w156:i32)  [unwired: 11 in]
          n95 = call "BRig_dataLC_Cue2_First_Prob_l2.vi"() -> ("output_Cue2_First_Prob_l2"=w155:i32)  [unwired: 11 in]
          n96 = call "BRig_dataLC_Cue2_First_Delay_l2.vi"() -> ("output_Cue2_First_Delay_l2"=w154:i32)  [unwired: 11 in]
          n97 = call "BRig_dataLC_Cue2_First_DelayOpt_l2.vi"() -> ("output_Cue2_First_DelayOpt_l2"=w153:i32)  [unwired: 11 in]
          n98 = call "BRig_dataLC_Cue2_First_Count_l2.vi"() -> ("output_Cue2_First_Count_l2"=w152:i32)  [unwired: 11 in]
          n99 = call "BRig_dataLC_Cue2_PostR_OnOff_l2.vi"() -> ("output_Cue2_PostR_OnOff_l2"=w151:i32)  [unwired: 11 in]
          n100 = call "BRig_dataLC_Cue2_PostR_Block_l2.vi"() -> ("output_Cue2_PostR_Block_l2"=w150:i32)  [unwired: 11 in]
          n101 = call "BRig_dataLC_Cue2_PostR_Prob_l2.vi"() -> ("output_Cue2_PostR_Prob_l2"=w149:i32)  [unwired: 11 in]
          n102 = call "BRig_dataLC_Cue2_PostR_Delay_l2.vi"() -> ("output_Cue2_PostR_Delay_l2"=w148:i32)  [unwired: 11 in]
          n103 = call "BRig_dataLC_Cue2_PostR_DelayOpt_l2.vi"() -> ("output_Cue2_PostR_DelayOpt_l2"=w147:i32)  [unwired: 11 in]
          n104 = call "BRig_dataLC_Cue2_PostR_Count_l2.vi"() -> ("output_Cue2_PostR_Count_l2"=w146:i32)  [unwired: 11 in]
          n105 = call "BRig_dataLC_Cue2_PreR_OnOff_l2.vi"() -> ("output_Cue2_PreR_OnOff_l2"=w145:i32)  [unwired: 11 in]
          n106 = call "BRig_dataLC_Cue2_PreR_Block_l2.vi"() -> ("output_Cue2_PreR_Block_l2"=w144:i32)  [unwired: 11 in]
          n107 = call "BRig_dataLC_Cue2_PreR_Prob_l2.vi"() -> ("output_Cue2_PreR_Prob_l2"=w143:i32)  [unwired: 11 in]
          n108 = call "BRig_dataLC_Cue2_PreR_Delay_l2.vi"() -> ("output_Cue2_PreR_Delay_l2"=w142:i32)  [unwired: 11 in]
          n109 = call "BRig_dataLC_Cue2_PreR_DelayOpt_l2.vi"() -> ("output_Cue2_PreR_DelayOpt_l2"=w141:i32)  [unwired: 11 in]
          n110 = call "BRig_dataLC_Cue2_PreR_Count_l2.vi"() -> ("output_Cue2_PreR_Count_l2"=w140:i32)  [unwired: 11 in]
          n111 = Boolean To (0,1)(Boolean="LC_Cue_First_OnOff") -> (0, 1=w232:i16)
          n112 = Boolean To (0,1)(Boolean="LC_Cue_First_delayOpt") -> (0, 1=w231:i16)
          n113 = Boolean To (0,1)(Boolean="LC_Cue_PreR_OnOff") -> (0, 1=w230:i16)
          n114 = Boolean To (0,1)(Boolean="LC_Cue_PreR_delayOpt") -> (0, 1=w229:i16)
          n115 = Boolean To (0,1)(Boolean="LC_Cue_PostR_OnOff") -> (0, 1=w228:i16)
          n116 = Boolean To (0,1)(Boolean="LC_Cue_PostR_delayOpt") -> (0, 1=w227:i16)
          n117 = Boolean To (0,1)(Boolean="LC_Cue2_First_OnOff") -> (0, 1=w205:i16)
          n118 = Boolean To (0,1)(Boolean="LC_Cue2_First_delayOpt") -> (0, 1=w204:i16)
          n119 = Boolean To (0,1)(Boolean="LC_Cue2_PreR_OnOff") -> (0, 1=w203:i16)
          n120 = Boolean To (0,1)(Boolean="LC_Cue2_PreR_delayOpt") -> (0, 1=w202:i16)
          n121 = Boolean To (0,1)(Boolean="LC_Cue2_PostR_OnOff") -> (0, 1=w201:i16)
          n122 = Boolean To (0,1)(Boolean="LC_Cue2_PostR_delayOpt") -> (0, 1=w200:i16)
          n123 = To Unsigned Word Integer(number=w232) -> (unsigned 16bit integer=w226:u16)
          n124 = To Unsigned Word Integer(number=w231) -> (unsigned 16bit integer=w222:u16)
          n125 = To Unsigned Word Integer(number=w230) -> (unsigned 16bit integer=w220:u16)
          n126 = To Unsigned Word Integer(number=w229) -> (unsigned 16bit integer=w216:u16)
          n127 = To Unsigned Word Integer(number=w228) -> (unsigned 16bit integer=w214:u16)
          n128 = To Unsigned Word Integer(number=w227) -> (unsigned 16bit integer=w210:u16)
          n129 = To Unsigned Word Integer(number=w205) -> (unsigned 16bit integer=w193:u16)
          n130 = To Unsigned Word Integer(number=w204) -> (unsigned 16bit integer=w189:u16)
          n131 = To Unsigned Word Integer(number=w203) -> (unsigned 16bit integer=w187:u16)
          n132 = To Unsigned Word Integer(number=w202) -> (unsigned 16bit integer=w183:u16)
          n133 = To Unsigned Word Integer(number=w201) -> (unsigned 16bit integer=w181:u16)
          n134 = To Unsigned Word Integer(number=w200) -> (unsigned 16bit integer=w177:u16)
          n135 = call "BRig_dataLC_Cue_PostR_nRew1_l2.vi"() -> ("output_Cue_PostR_nRew1_l2"=w139:i32)  [unwired: 11 in]
          n136 = call "BRig_dataLC_Cue_PostR_nRew2_l2.vi"() -> ("output_Cue_PostR_nRew2_l2"=w138:i32)  [unwired: 11 in]
          n137 = call "BRig_dataLC_Cue2_PostR_nRew1_l2.vi"() -> ("output_Cue2_PostR_nRew1_l2"=w137:i32)  [unwired: 11 in]
          n138 = call "BRig_dataLC_Cue2_PostR_nRew2_l2.vi"() -> ("output_Cue2_PostR_nRew2_l2"=w136:i32)  [unwired: 11 in]
          n139 = Replace Array Subset(array=w240, new element #1=w207, index #1=w208, new element #2=w226, index #2=w158, new element #3="LC_Cue_First_Block", index #3=w159, new element #4="LC_Cue_First_Probability", index #4=w160, new element #5="LC_Cue_First_Tdelay", index #5=w161, new element #6=w222, index #6=w162, new element #7="LC_Cue_First_Count", index #7=w163, new element #8=w220, index #8=w164, new element #9="LC_Cue_PreR_Block", index #9=w165, new element #10="LC_Cue_PreR_Probability", index #10=w166, new element #11="LC_Cue_PreR_Tdelay", index #11=w167, new element #12=w216, index #12=w168, new element #13="LC_Cue_PreR_Count", index #13=w169, new element #14=w214, index #14=w170, new element #15="LC_Cue_PostR_Block", index #15=w171, new element #16="LC_Cue_PostR_Probability", index #16=w172, new element #17="LC_Cue_PostR_Tdelay", index #17=w173, new element #18=w210, index #18=w174, new element #19="LC_Cue_PostR_Count", index #19=w175, new element #20=w193, index #20=w157, new element #21="LC_Cue2_First_Block", index #21=w156, new element #22="LC_Cue2_First_Probability", index #22=w155, new element #23="LC_Cue2_First_Tdelay", index #23=w154, new element #24=w189, index #24=w153, new element #25="LC_Cue2_First_Count", index #25=w152, new element #26=w187, index #26=w151, new element #27="LC_Cue2_PreR_Block", index #27=w150, new element #28="LC_Cue2_PreR_Probability", index #28=w149, new element #29="LC_Cue2_PreR_Tdelay", index #29=w148, new element #30=w183, index #30=w147, new element #31="LC_Cue2_PreR_Count", index #31=w146, new element #32=w181, index #32=w145, new element #33="LC_Cue2_PostR_Block", index #33=w144, new element #34="LC_Cue2_PostR_Probability", index #34=w143, new element #35="LC_Cue2_PostR_Tdelay", index #35=w142, new element #36=w177, index #36=w141, new element #37="LC_Cue2_PostR_Count", index #37=w140, new element #38="LC_Cue_nRew1", index #38=w139, new element #39="LC_Cue_nRew2", index #39=w138, new element #40="LC_Cue2_nRew1", index #40=w137, new element #41="LC_Cue2_nRew2", index #41=w136) -> (w239:u16[])
        }
        frame 3 {
          n140 = call "BRig_dataLC_Selection_First_OnOff_l2.vi"() -> ("output_Selection_First_OnOff_l2"=w245:i32)  [unwired: 11 in]
          n141 = call "BRig_dataLC_Selection_First_Block_l2.vi"() -> ("output_Selection_First_Block_l2"=w246:i32)  [unwired: 11 in]
          n142 = call "BRig_dataLC_Selection_First_Prob_l2.vi"() -> ("output_Selection_First_Prob_l2"=w247:i32)  [unwired: 11 in]
          n143 = call "BRig_dataLC_Selection_First_Delay_l2.vi"() -> ("output_Selection_First_Delay_l2"=w248:i32)  [unwired: 11 in]
          n144 = call "BRig_dataLC_Selection_First_Count_l2.vi"() -> ("output_Selection_First_Count_l2"=w249:i32)  [unwired: 11 in]
          n145 = call "BRig_dataLC_Selection_PreR_OnOff_l2.vi"() -> ("output_Selection_PreR_OnOff_l2"=w250:i32)  [unwired: 11 in]
          n146 = call "BRig_dataLC_Selection_PreR_Block_l2.vi"() -> ("output_Selection_PreR_Block_l2"=w251:i32)  [unwired: 11 in]
          n147 = call "BRig_dataLC_Selection_PreR_Prob_l2.vi"() -> ("output_Selection_PreR_Prob_l2"=w252:i32)  [unwired: 11 in]
          n148 = call "BRig_dataLC_Selection_PreR_Delay_l2.vi"() -> ("output_Selection_PreR_Delay_l2"=w253:i32)  [unwired: 11 in]
          n149 = call "BRig_dataLC_Selection_PreR_Count_l2.vi"() -> ("output_Selection_PreR_Count_l2"=w254:i32)  [unwired: 11 in]
          n150 = call "BRig_dataLC_Selection_PostR_OnOff_l2.vi"() -> ("output_Selection_PostR_OnOff_l2"=w255:i32)  [unwired: 11 in]
          n151 = call "BRig_dataLC_Selection_PostR_Block_l2.vi"() -> ("output_Selection_PostR_Block_l2"=w256:i32)  [unwired: 11 in]
          n152 = call "BRig_dataLC_Selection_PostR_Prob_l2.vi"() -> ("output_Selection_PostR_Prob_l2"=w257:i32)  [unwired: 11 in]
          n153 = call "BRig_dataLC_Selection_PostR_Delay_l2.vi"() -> ("output_Selection_PostR_Delay_l2"=w258:i32)  [unwired: 11 in]
          n154 = call "BRig_dataLC_Selection_PostR_Count_l2.vi"() -> ("output_Selection_PostR_Count_l2"=w259:i32)  [unwired: 11 in]
          n155 = Boolean To (0,1)(Boolean="LC_Sel_First_OnOff") -> (0, 1=w280:i16)
          n156 = Boolean To (0,1)(Boolean="LC_Sel_PreR_OnOff") -> (0, 1=w279:i16)
          n157 = Boolean To (0,1)(Boolean="LC_Sel_PostR_OnOff") -> (0, 1=w278:i16)
          n158 = To Unsigned Word Integer(number=w280) -> (unsigned 16bit integer=w277:u16)
          n159 = To Unsigned Word Integer(number=w279) -> (unsigned 16bit integer=w272:u16)
          n160 = To Unsigned Word Integer(number=w278) -> (unsigned 16bit integer=w267:u16)
          n161 = call "BRig_dataLC_Selection_PostR_nRew1_l2.vi"() -> ("output_Selection_PostR_nRew1_l2"=w244:i32)  [unwired: 11 in]
          n162 = call "BRig_dataLC_Selection_PostR_nRew2_l2.vi"() -> ("output_Selection_PostR_nRew2_l2"=w243:i32)  [unwired: 11 in]
          n163 = Replace Array Subset(array=w285, new element #1=w261, index #1=w262, new element #2=w277, index #2=w245, new element #3="LC_Sel_First_Block", index #3=w246, new element #4="LC_Sel_First_Probability", index #4=w247, new element #5="LC_Sel_First_Tdelay", index #5=w248, new element #6="LC_Sel_First_Count", index #6=w249, new element #7=w272, index #7=w250, new element #8="LC_Sel_PreR_Block", index #8=w251, new element #9="LC_Sel_PreR_Probability", index #9=w252, new element #10="LC_Sel_PreR_Tdelay", index #10=w253, new element #11="LC_Sel_PreR_Count", index #11=w254, new element #12=w267, index #12=w255, new element #13="LC_Sel_PostR_Block", index #13=w256, new element #14="LC_Sel_PostR_Probability", index #14=w257, new element #15="LC_Sel_PostR_Tdelay", index #15=w258, new element #16="LC_Sel_PostR_Count", index #16=w259, new element #17="LC_Sel_nRew1", index #17=w244, new element #18="LC_Sel_nRew2", index #18=w243) -> (w284:u16[])
        }
        frame 4 {
          n164 = call "BRig_dataLC_Reward_OnOff_l2.vi"() -> ("output_Reward_OnOff_l2"=w294:i32)  [unwired: 11 in]
          n165 = call "BRig_dataLC_Reward_Block_l2.vi"() -> ("output_Reward_Block_l2"=w295:i32)  [unwired: 11 in]
          n166 = call "BRig_dataLC_Reward_Trial_l2.vi"() -> ("output_Reward_Trial_l2"=w296:i32)  [unwired: 11 in]
          n167 = call "BRig_dataLC_Reward_Prob_l2.vi"() -> ("output_Reward_Prob_l2"=w297:i32)  [unwired: 11 in]
          n168 = call "BRig_dataLC_Reward_Delay_l2.vi"() -> ("output_Reward_Delay_l2"=w298:i32)  [unwired: 11 in]
          n169 = call "BRig_dataLC_Wrong_OnOff_l2.vi"() -> ("output_Wrong_OnOff_l2"=w299:i32)  [unwired: 11 in]
          n170 = call "BRig_dataLC_Wrong_Block_l2.vi"() -> ("output_Wrong_Block_l2"=w300:i32)  [unwired: 11 in]
          n171 = call "BRig_dataLC_Wrong_Trial_l2.vi"() -> ("output_Wrong_Trial_l2"=w301:i32)  [unwired: 11 in]
          n172 = call "BRig_dataLC_Wrong_Prob_l2.vi"() -> ("output_Wrong_Prob_l2"=w302:i32)  [unwired: 11 in]
          n173 = call "BRig_dataLC_Wrong_Delay_l2.vi"() -> ("output_Wrong_Delay_l2"=w303:i32)  [unwired: 11 in]
          n174 = Boolean To (0,1)(Boolean="LC_Reward_OnOff") -> (0, 1=w318:i16)
          n175 = Boolean To (0,1)(Boolean="LC_Wrong_OnOff") -> (0, 1=w317:i16)
          n176 = To Unsigned Word Integer(number=w318) -> (unsigned 16bit integer=w316:u16)
          n177 = To Unsigned Word Integer(number=w317) -> (unsigned 16bit integer=w311:u16)
          n178 = call "BRig_dataLC_Reward_nRew1_l2.vi"() -> ("output_Reward_nRew1_l2"=w290:i32)  [unwired: 11 in]
          n179 = call "BRig_dataLC_Reward_nRew2_l2.vi"() -> ("output_Reward_nRew2_l2"=w291:i32)  [unwired: 11 in]
          n180 = call "BRig_dataLC_Wrong_nRew1_l2.vi"() -> ("output_Wrong_nRew1_l2"=w289:i32)  [unwired: 11 in]
          n181 = call "BRig_dataLC_Wrong_nRew2_l2.vi"() -> ("output_Wrong_nRew2_l2"=w287:i32)  [unwired: 11 in]
          n182 = Replace Array Subset(array=w322, new element #1=w305, index #1=w306, new element #2=w316, index #2=w294, new element #3="LC_Reward_Block", index #3=w295, new element #4="LC_Reward_Trial", index #4=w296, new element #5="LC_Reward_Probability", index #5=w297, new element #6="LC_Reward_Tdelay", index #6=w298, new element #7=w311, index #7=w299, new element #8="LC_Wrong_Block", index #8=w300, new element #9="LC_Wrong_Trial", index #9=w301, new element #10="LC_Wrong_Probability", index #10=w302, new element #11="LC_Wrong_Tdelay", index #11=w303, new element #12="LC_Rew_nRew1", index #12=w290, new element #13="LC_Rew_nRew2", index #13=w291, new element #14="LC_Wro_nRew1", index #14=w289, new element #15="LC_Wro_nRew2", index #15=w287) -> (w321:u16[])
        }
        frame 5 {
          w346 = 100.0 ("y")
          n183 = call "BRig_dataExp_LED_baseline_l2.vi"() -> ("output_LED_baseline_l2"=w323:i32)  [unwired: 11 in]
          n184 = call "BRig_dataExp_L_freq_l2.vi"() -> ("output_L_freq_l2"=w324:i32)  [unwired: 11 in]
          n185 = call "BRig_dataExp_L_T_l2.vi"() -> ("output_L_T_l2"=w325:i32)  [unwired: 11 in]
          n186 = call "BRig_dataExp_L_Tpeak_l2.vi"() -> ("output_L_Tpeak_l2"=w326:i32)  [unwired: 11 in]
          n187 = call "BRig_dataExp_L_Tshutter_l2.vi"() -> ("output_L_Tshutter_l2"=w327:i32)  [unwired: 11 in]
          n188 = call "BRig_dataExp_L_power_min_l2.vi"() -> ("output_L_power_min_l2"=w328:i32)  [unwired: 11 in]
          n189 = call "BRig_dataExp_L_power_max_l2.vi"() -> ("output_L_power_max_l2"=w329:i32)  [unwired: 11 in]
          n190 = call "BRig_dataExp_L_power_step_l2.vi"() -> ("output_L_power_step_l2"=w330:i32)  [unwired: 11 in]
          n191 = call "BRig_dataExp_L_Ttotal_l2.vi"() -> ("output_L_Ttotal_l2"=w331:i32)  [unwired: 11 in]
          n192 = Boolean To (0,1)(Boolean="LED_baseline") -> (0, 1=w358:i16)
          n193 = To Unsigned Word Integer(number=w358) -> (unsigned 16bit integer=w356:u16)
          n194 = Multiply(x="Laser_power_min", y=w346) -> (x*y=w350:dbl)
          n195 = Multiply(x="Laser_power_max", y=w346) -> (x*y=w352:dbl)
          n196 = Multiply(x="Laser_power_step", y=w346) -> (x*y=w355:dbl)
          n197 = Round To Nearest(number=w350) -> (nearest integer value=w349:dbl)
          n198 = Round To Nearest(number=w352) -> (nearest integer value=w351:dbl)
          n199 = Round To Nearest(number=w355) -> (nearest integer value=w354:dbl)
          n200 = To Unsigned Word Integer(number=w349) -> (unsigned 16bit integer=w343:u16)
          n201 = To Unsigned Word Integer(number=w351) -> (unsigned 16bit integer=w344:u16)
          n202 = To Unsigned Word Integer(number=w354) -> (unsigned 16bit integer=w345:u16)
          n203 = Add(x="Laser_T", y="Laser_Tshutter") -> (x+y=w338:u16)
          n204 = Replace Array Subset(array=w335, new element=w332, index=w333) -> (w334:u16[])
          n205 = Replace Array Subset(array=w337, new element #1=w356, index #1=w323, new element #2="Laser_Freq", index #2=w324, new element #3="Laser_T", index #3=w325, new element #4="Laser_Tpeak", index #4=w326, new element #5="Laser_Tshutter", index #5=w327, new element #6=w343, index #6=w328, new element #7=w344, index #7=w329, new element #8=w345, index #8=w330, new element #9=w338, index #9=w331) -> (w336:u16[])
        }
        frame 6 {
          n206 = call "BRig_dataExp_L_freq_l2.vi"() -> ("output_L_freq_l2"=w359:i32)  [unwired: 11 in]
          n207 = call "BRig_dataExp_L_T_l2.vi"() -> ("output_L_T_l2"=w360:i32)  [unwired: 11 in]
          n208 = call "BRig_dataExp_L_Tpeak_l2.vi"() -> ("output_L_Tpeak_l2"=w361:i32)  [unwired: 11 in]
          n209 = call "BRig_dataExp_L_Tshutter_l2.vi"() -> ("output_L_Tshutter_l2"=w362:i32)  [unwired: 11 in]
          n210 = Replace Array Subset(array=w366, new element=w363, index=w364) -> (w365:u16[])
          n211 = call "BRig_RT__Case_Idle__calc_LaserPulse.vi"("input_dataExp_L_Tshutter"=w362, "input_dataExp_L_Tpeak"=w361, "input_dataExp_L_T"=w360, "input_dataExp_L_freq"=w359, "input_dataExp"=w368) -> ("output_cluster"=→"LaserPulseTrain":cluster{u16[], u16[]})  [unwired: 6 in]
        }
      }
    }
    frame True {
      w533 = 100.0 ("y")
      n212 = call "BRig_dataLC_ENL_First_OnOff_l2.vi"() -> ("output_ENL_First_OnOff_l2"=w466:i32)  [unwired: 11 in]
      n213 = call "BRig_dataLC_ENL_First_Block_l2.vi"() -> ("output_ENL_First_Block_l2"=w465:i32)  [unwired: 11 in]
      n214 = call "BRig_dataLC_ENL_First_Prob_l2.vi"() -> ("output_ENL_First_Prob_l2"=w467:i32)  [unwired: 11 in]
      n215 = call "BRig_dataLC_ENL_First_Delay_l2.vi"() -> ("output_ENL_First_Delay_l2"=w468:i32)  [unwired: 11 in]
      n216 = call "BRig_dataLC_ENL_First_DelayOpt_l2.vi"() -> ("output_ENL_First_DelayOpt_l2"=w469:i32)  [unwired: 11 in]
      n217 = call "BRig_dataLC_ENL_First_Count_l2.vi"() -> ("output_ENL_First_Count_l2"=w470:i32)  [unwired: 11 in]
      n218 = call "BRig_dataLC_ENL_PreR_OnOff_l2.vi"() -> ("output_ENL_PreR_OnOff_l2"=w471:i32)  [unwired: 11 in]
      n219 = call "BRig_dataLC_ENL_PreR_Block_l2.vi"() -> ("output_ENL_PreR_Block_l2"=w472:i32)  [unwired: 11 in]
      n220 = call "BRig_dataLC_ENL_PreR_Prob_l2.vi"() -> ("output_ENL_PreR_Prob_l2"=w473:i32)  [unwired: 11 in]
      n221 = call "BRig_dataLC_ENL_PreR_Delay_l2.vi"() -> ("output_ENL_PreR_Delay_l2"=w474:i32)  [unwired: 11 in]
      n222 = call "BRig_dataLC_ENL_PreR_DelayOpt_l2.vi"() -> ("output_ENL_PreR_DelayOpt_l2"=w475:i32)  [unwired: 11 in]
      n223 = call "BRig_dataLC_ENL_PreR_Count_l2.vi"() -> ("output_ENL_PreR_Count_l2"=w476:i32)  [unwired: 11 in]
      n224 = call "BRig_dataLC_ENL_PostR_OnOff_l2.vi"() -> ("output_ENL_PostR_OnOff_l2"=w477:i32)  [unwired: 11 in]
      n225 = call "BRig_dataLC_ENL_PostR_Block_l2.vi"() -> ("output_ENL_PostR_Block_l2"=w478:i32)  [unwired: 11 in]
      n226 = call "BRig_dataLC_ENL_PostR_Prob_l2.vi"() -> ("output_ENL_PostR_Prob_l2"=w479:i32)  [unwired: 11 in]
      n227 = call "BRig_dataLC_ENL_PostR_Delay_l2.vi"() -> ("output_ENL_PostR_Delay_l2"=w480:i32)  [unwired: 11 in]
      n228 = call "BRig_dataLC_ENL_PostR_DelayOpt_l2.vi"() -> ("output_ENL_PostR_DelayOpt_l2"=w481:i32)  [unwired: 11 in]
      n229 = call "BRig_dataLC_ENL_PostR_Count_l2.vi"() -> ("output_ENL_PostR_Count_l2"=w482:i32)  [unwired: 11 in]
      n230 = call "BRig_dataLC_Reward_nRew1_l2.vi"() -> ("output_Reward_nRew1_l2"=w376:i32)  [unwired: 11 in]
      n231 = call "BRig_dataLC_Reward_nRew2_l2.vi"() -> ("output_Reward_nRew2_l2"=w375:i32)  [unwired: 11 in]
      n232 = call "BRig_dataLC_Wrong_nRew1_l2.vi"() -> ("output_Wrong_nRew1_l2"=w372:i32)  [unwired: 11 in]
      n233 = call "BRig_dataLC_Wrong_nRew2_l2.vi"() -> ("output_Wrong_nRew2_l2"=w371:i32)  [unwired: 11 in]
      n234 = call "BRig_dataLC_ENL2_First_OnOff_l2.vi"() -> ("output_ENL2_First_OnOff_l2"=w401:i32)  [unwired: 11 in]
      n235 = call "BRig_dataLC_ENL2_First_Block_l2.vi"() -> ("output_ENL2_First_Block_l2"=w400:i32)  [unwired: 11 in]
      n236 = call "BRig_dataLC_ENL2_First_Prob_l2.vi"() -> ("output_ENL2_First_Prob_l2"=w399:i32)  [unwired: 11 in]
      n237 = call "BRig_dataLC_ENL2_First_Delay_l2.vi"() -> ("output_ENL2_First_Delay_l2"=w398:i32)  [unwired: 11 in]
      n238 = call "BRig_dataLC_ENL2_First_DelayOpt_l2.vi"() -> ("output_ENL2_First_DelayOpt_l2"=w397:i32)  [unwired: 11 in]
      n239 = call "BRig_dataLC_ENL2_First_Count_l2.vi"() -> ("output_ENL2_First_Count_l2"=w396:i32)  [unwired: 11 in]
      n240 = call "BRig_dataLC_ENL2_PreR_OnOff_l2.vi"() -> ("output_ENL2_PreR_OnOff_l2"=w407:i32)  [unwired: 11 in]
      n241 = call "BRig_dataLC_ENL2_PreR_Block_l2.vi"() -> ("output_ENL2_PreR_Block_l2"=w406:i32)  [unwired: 11 in]
      n242 = call "BRig_dataLC_ENL2_PreR_Prob_l2.vi"() -> ("output_ENL2_PreR_Prob_l2"=w405:i32)  [unwired: 11 in]
      n243 = call "BRig_dataLC_ENL2_PreR_Delay_l2.vi"() -> ("output_ENL2_PreR_Delay_l2"=w404:i32)  [unwired: 11 in]
      n244 = call "BRig_dataLC_ENL2_PreR_DelayOpt_l2.vi"() -> ("output_ENL2_PreR_DelayOpt_l2"=w403:i32)  [unwired: 11 in]
      n245 = call "BRig_dataLC_ENL2_PreR_Count_l2.vi"() -> ("output_ENL2_PreR_Count_l2"=w402:i32)  [unwired: 11 in]
      n246 = call "BRig_dataLC_ENL2_PostR_OnOff_l2.vi"() -> ("output_ENL2_PostR_OnOff_l2"=w413:i32)  [unwired: 11 in]
      n247 = call "BRig_dataLC_ENL2_PostR_Block_l2.vi"() -> ("output_ENL2_PostR_Block_l2"=w412:i32)  [unwired: 11 in]
      n248 = call "BRig_dataLC_ENL2_PostR_Prob_l2.vi"() -> ("output_ENL2_PostR_Prob_l2"=w411:i32)  [unwired: 11 in]
      n249 = call "BRig_dataLC_ENL2_PostR_Delay_l2.vi"() -> ("output_ENL2_PostR_Delay_l2"=w410:i32)  [unwired: 11 in]
      n250 = call "BRig_dataLC_ENL2_PostR_DelayOpt_l2.vi"() -> ("output_ENL2_PostR_DelayOpt_l2"=w409:i32)  [unwired: 11 in]
      n251 = call "BRig_dataLC_ENL2_PostR_Count_l2.vi"() -> ("output_ENL2_PostR_Count_l2"=w408:i32)  [unwired: 11 in]
      n252 = Index Array(array=w377, index #1=w376, index #2=w375, index #3=w372, index #4=w371) -> (element #1=w374:u16, element #2=w373:u16, element #3=w370:u16, element #4=w369:u16)
      n253 = Index Array(array=w547, index #1=w466, index #2=w465, index #3=w467, index #4=w468, index #5=w469, index #6=w470, index #7=w471, index #8=w472, index #9=w473, index #10=w474, index #11=w475, index #12=w476, index #13=w477, index #14=w478, index #15=w479, index #16=w480, index #17=w481, index #18=w482) -> (element #1=w619:u16, element #2=w618:u16, element #3=w617:u16, element #4=w616:u16, element #5=w615:u16, element #6=w614:u16, element #7=w613:u16, element #8=w612:u16, element #9=w611:u16, element #10=w610:u16, element #11=w609:u16, element #12=w608:u16, element #13=w607:u16, element #14=w606:u16, element #15=w605:u16, element #16=w604:u16, element #17=w603:u16, element #18=w602:u16)
      n254 = local write "LC_Rew_nRew1"(w374) -> ()
      n255 = local write "LC_Rew_nRew2"(w373) -> ()
      n256 = local write "LC_Wro_nRew1"(w370) -> ()
      n257 = local write "LC_Wro_nRew2"(w369) -> ()
      n258 = Index Array(array=w377, index #1=w401, index #2=w400, index #3=w399, index #4=w398, index #5=w397, index #6=w396, index #7=w407, index #8=w406, index #9=w405, index #10=w404, index #11=w403, index #12=w402, index #13=w413, index #14=w412, index #15=w411, index #16=w410, index #17=w409, index #18=w408) -> (element #1=w507:u16, element #2=w508:u16, element #3=w509:u16, element #4=w510:u16, element #5=w511:u16, element #6=w512:u16, element #7=w513:u16, element #8=w514:u16, element #9=w515:u16, element #10=w516:u16, element #11=w517:u16, element #12=w518:u16, element #13=w520:u16, element #14=w521:u16, element #15=w522:u16, element #16=w523:u16, element #17=w524:u16, element #18=w525:u16)
      n259 = Not Equal To 0?(x=w619) -> (x != 0?=w625:bool)
      n260 = Not Equal To 0?(x=w615) -> (x != 0?=w624:bool)
      n261 = Not Equal To 0?(x=w613) -> (x != 0?=w623:bool)
      n262 = Not Equal To 0?(x=w609) -> (x != 0?=w622:bool)
      n263 = Not Equal To 0?(x=w607) -> (x != 0?=w621:bool)
      n264 = Not Equal To 0?(x=w603) -> (x != 0?=w620:bool)
      n265 = local write "LC_ENL_First_OnOff"(w625) -> ()
      n266 = local write "LC_ENL_First_Block"(w618) -> ()
      n267 = local write "LC_ENL_First_Probability"(w617) -> ()
      n268 = local write "LC_ENL_First_Tdelay"(w616) -> ()
      n269 = local write "LC_ENL_First_delayOpt"(w624) -> ()
      n270 = local write "LC_ENL_First_Count"(w614) -> ()
      n271 = local write "LC_ENL_PreR_OnOff"(w623) -> ()
      n272 = local write "LC_ENL_PreR_Block"(w612) -> ()
      n273 = local write "LC_ENL_PreR_Probability"(w611) -> ()
      n274 = local write "LC_ENL_PreR_Tdelay"(w610) -> ()
      n275 = local write "LC_ENL_PreR_delayOpt"(w622) -> ()
      n276 = local write "LC_ENL_PreR_Count"(w608) -> ()
      n277 = local write "LC_ENL_PostR_OnOff"(w621) -> ()
      n278 = local write "LC_ENL_PostR_Block"(w606) -> ()
      n279 = local write "LC_ENL_PostR_Probability"(w605) -> ()
      n280 = local write "LC_ENL_PostR_Tdelay"(w604) -> ()
      n281 = local write "LC_ENL_PostR_delayOpt"(w620) -> ()
      n282 = local write "LC_ENL_PostR_Count"(w602) -> ()
      n283 = Not Equal To 0?(x=w507) -> (x != 0?=w528:bool)
      n284 = Not Equal To 0?(x=w511) -> (x != 0?=w529:bool)
      n285 = Not Equal To 0?(x=w513) -> (x != 0?=w527:bool)
      n286 = Not Equal To 0?(x=w517) -> (x != 0?=w530:bool)
      n287 = Not Equal To 0?(x=w520) -> (x != 0?=w526:bool)
      n288 = Not Equal To 0?(x=w524) -> (x != 0?=w519:bool)
      n289 = local write "LC_ENL2_First_OnOff"(w528) -> ()
      n290 = local write "LC_ENL2_First_Block"(w508) -> ()
      n291 = local write "LC_ENL2_First_Probability"(w509) -> ()
      n292 = local write "LC_ENL2_First_Tdelay"(w510) -> ()
      n293 = local write "LC_ENL2_First_delayOpt"(w529) -> ()
      n294 = local write "LC_ENL2_First_Count"(w512) -> ()
      n295 = local write "LC_ENL2_PreR_OnOff"(w527) -> ()
      n296 = local write "LC_ENL2_PreR_Block"(w514) -> ()
      n297 = local write "LC_ENL2_PreR_Probability"(w515) -> ()
      n298 = local write "LC_ENL2_PreR_Tdelay"(w516) -> ()
      n299 = local write "LC_ENL2_PreR_delayOpt"(w530) -> ()
      n300 = local write "LC_ENL2_PreR_Count"(w518) -> ()
      n301 = local write "LC_ENL2_PostR_OnOff"(w526) -> ()
      n302 = local write "LC_ENL2_PostR_Block"(w521) -> ()
      n303 = local write "LC_ENL2_PostR_Probability"(w522) -> ()
      n304 = local write "LC_ENL2_PostR_Tdelay"(w523) -> ()
      n305 = local write "LC_ENL2_PostR_delayOpt"(w519) -> ()
      n306 = local write "LC_ENL2_PostR_Count"(w525) -> ()
      n307 = call "BRig_dataLC_Cue_First_OnOff_l2.vi"() -> ("output_Cue_First_OnOff_l2"=w449:i32)  [unwired: 11 in]
      n308 = call "BRig_dataLC_Cue_First_Block_l2.vi"() -> ("output_Cue_First_Block_l2"=w447:i32)  [unwired: 11 in]
      n309 = call "BRig_dataLC_Cue_First_Prob_l2.vi"() -> ("output_Cue_First_Prob_l2"=w448:i32)  [unwired: 11 in]
      n310 = call "BRig_dataLC_Cue_First_Delay_l2.vi"() -> ("output_Cue_First_Delay_l2"=w450:i32)  [unwired: 11 in]
      n311 = call "BRig_dataLC_Cue_First_DelayOpt_l2.vi"() -> ("output_Cue_First_DelayOpt_l2"=w451:i32)  [unwired: 11 in]
      n312 = call "BRig_dataLC_Cue_First_Count_l2.vi"() -> ("output_Cue_First_Count_l2"=w452:i32)  [unwired: 11 in]
      n313 = call "BRig_dataLC_Cue_PreR_OnOff_l2.vi"() -> ("output_Cue_PreR_OnOff_l2"=w453:i32)  [unwired: 11 in]
      n314 = call "BRig_dataLC_Cue_PreR_Block_l2.vi"() -> ("output_Cue_PreR_Block_l2"=w454:i32)  [unwired: 11 in]
      n315 = call "BRig_dataLC_Cue_PreR_Prob_l2.vi"() -> ("output_Cue_PreR_Prob_l2"=w455:i32)  [unwired: 11 in]
      n316 = call "BRig_dataLC_Cue_PreR_Delay_l2.vi"() -> ("output_Cue_PreR_Delay_l2"=w456:i32)  [unwired: 11 in]
      n317 = call "BRig_dataLC_Cue_PreR_DelayOpt_l2.vi"() -> ("output_Cue_PreR_DelayOpt_l2"=w457:i32)  [unwired: 11 in]
      n318 = call "BRig_dataLC_Cue_PreR_Count_l2.vi"() -> ("output_Cue_PreR_Count_l2"=w458:i32)  [unwired: 11 in]
      n319 = call "BRig_dataLC_Cue_PostR_OnOff_l2.vi"() -> ("output_Cue_PostR_OnOff_l2"=w459:i32)  [unwired: 11 in]
      n320 = call "BRig_dataLC_Cue_PostR_Block_l2.vi"() -> ("output_Cue_PostR_Block_l2"=w460:i32)  [unwired: 11 in]
      n321 = call "BRig_dataLC_Cue_PostR_Prob_l2.vi"() -> ("output_Cue_PostR_Prob_l2"=w461:i32)  [unwired: 11 in]
      n322 = call "BRig_dataLC_Cue_PostR_Delay_l2.vi"() -> ("output_Cue_PostR_Delay_l2"=w462:i32)  [unwired: 11 in]
      n323 = call "BRig_dataLC_Cue_PostR_DelayOpt_l2.vi"() -> ("output_Cue_PostR_DelayOpt_l2"=w463:i32)  [unwired: 11 in]
      n324 = call "BRig_dataLC_Cue_PostR_Count_l2.vi"() -> ("output_Cue_PostR_Count_l2"=w464:i32)  [unwired: 11 in]
      n325 = call "BRig_dataExp_LED_baseline_l2.vi"() -> ("output_LED_baseline_l2"=w421:i32)  [unwired: 11 in]
      n326 = call "BRig_dataExp_L_freq_l2.vi"() -> ("output_L_freq_l2"=w420:i32)  [unwired: 11 in]
      n327 = call "BRig_dataExp_L_T_l2.vi"() -> ("output_L_T_l2"=w419:i32)  [unwired: 11 in]
      n328 = call "BRig_dataExp_L_Tpeak_l2.vi"() -> ("output_L_Tpeak_l2"=w418:i32)  [unwired: 11 in]
      n329 = call "BRig_dataExp_L_Tshutter_l2.vi"() -> ("output_L_Tshutter_l2"=w417:i32)  [unwired: 11 in]
      n330 = call "BRig_dataExp_L_power_min_l2.vi"() -> ("output_L_power_min_l2"=w416:i32)  [unwired: 11 in]
      n331 = call "BRig_dataExp_L_power_max_l2.vi"() -> ("output_L_power_max_l2"=w415:i32)  [unwired: 11 in]
      n332 = call "BRig_dataExp_L_power_step_l2.vi"() -> ("output_L_power_step_l2"=w414:i32)  [unwired: 11 in]
      n333 = Index Array(array=w547, index #1=w449, index #2=w447, index #3=w448, index #4=w450, index #5=w451, index #6=w452, index #7=w453, index #8=w454, index #9=w455, index #10=w456, index #11=w457, index #12=w458, index #13=w459, index #14=w460, index #15=w461, index #16=w462, index #17=w463, index #18=w464) -> (element #1=w595:u16, element #2=w594:u16, element #3=w593:u16, element #4=w592:u16, element #5=w591:u16, element #6=w590:u16, element #7=w589:u16, element #8=w588:u16, element #9=w587:u16, element #10=w586:u16, element #11=w585:u16, element #12=w584:u16, element #13=w583:u16, element #14=w582:u16, element #15=w581:u16, element #16=w580:u16, element #17=w579:u16, element #18=w578:u16)
      n334 = Index Array(array=w377, index #1=w421, index #2=w420, index #3=w419, index #4=w418, index #5=w417, index #6=w416, index #7=w415, index #8=w414) -> (element #1=w546:u16, element #2=w544:u16, element #3=w543:u16, element #4=w542:u16, element #5=w541:u16, element #6=w540:u16, element #7=w539:u16, element #8=w538:u16)
      n335 = To Double Precision Float(number=w540) -> (double precision float=w537:dbl)
      n336 = To Double Precision Float(number=w539) -> (double precision float=w532:dbl)
      n337 = To Double Precision Float(number=w538) -> (double precision float=w531:dbl)
      n338 = Not Equal To 0?(x=w595) -> (x != 0?=w601:bool)
      n339 = Not Equal To 0?(x=w591) -> (x != 0?=w600:bool)
      n340 = Not Equal To 0?(x=w589) -> (x != 0?=w599:bool)
      n341 = Not Equal To 0?(x=w585) -> (x != 0?=w598:bool)
      n342 = Not Equal To 0?(x=w583) -> (x != 0?=w597:bool)
      n343 = Not Equal To 0?(x=w579) -> (x != 0?=w596:bool)
      n344 = Divide(x=w537, y=w533) -> (x/y=w536:dbl)
      n345 = Divide(x=w532, y=w533) -> (x/y=w535:dbl)
      n346 = Divide(x=w531, y=w533) -> (x/y=w534:dbl)
      n347 = local write "LC_Cue_First_OnOff"(w601) -> ()
      n348 = local write "LC_Cue_First_Block"(w594) -> ()
      n349 = local write "LC_Cue_First_Probability"(w593) -> ()
      n350 = local write "LC_Cue_First_Tdelay"(w592) -> ()
      n351 = local write "LC_Cue_First_delayOpt"(w600) -> ()
      n352 = local write "LC_Cue_First_Count"(w590) -> ()
      n353 = local write "LC_Cue_PreR_OnOff"(w599) -> ()
      n354 = local write "LC_Cue_PreR_Block"(w588) -> ()
      n355 = local write "LC_Cue_PreR_Probability"(w587) -> ()
      n356 = local write "LC_Cue_PreR_Tdelay"(w586) -> ()
      n357 = local write "LC_Cue_PreR_delayOpt"(w598) -> ()
      n358 = local write "LC_Cue_PreR_Count"(w584) -> ()
      n359 = local write "LC_Cue_PostR_OnOff"(w597) -> ()
      n360 = local write "LC_Cue_PostR_Block"(w582) -> ()
      n361 = local write "LC_Cue_PostR_Probability"(w581) -> ()
      n362 = local write "LC_Cue_PostR_Tdelay"(w580) -> ()
      n363 = local write "LC_Cue_PostR_delayOpt"(w596) -> ()
      n364 = local write "LC_Cue_PostR_Count"(w578) -> ()
      n365 = Not Equal To 0?(x=w546) -> (x != 0?=w545:bool)
      n366 = call "BRig_dataLC_Cue2_First_OnOff_l2.vi"() -> ("output_Cue2_First_OnOff_l2"=w395:i32)  [unwired: 11 in]
      n367 = call "BRig_dataLC_Cue2_First_Block_l2.vi"() -> ("output_Cue2_First_Block_l2"=w394:i32)  [unwired: 11 in]
      n368 = call "BRig_dataLC_Cue2_First_Prob_l2.vi"() -> ("output_Cue2_First_Prob_l2"=w393:i32)  [unwired: 11 in]
      n369 = call "BRig_dataLC_Cue2_First_Delay_l2.vi"() -> ("output_Cue2_First_Delay_l2"=w392:i32)  [unwired: 11 in]
      n370 = call "BRig_dataLC_Cue2_First_DelayOpt_l2.vi"() -> ("output_Cue2_First_DelayOpt_l2"=w391:i32)  [unwired: 11 in]
      n371 = call "BRig_dataLC_Cue2_First_Count_l2.vi"() -> ("output_Cue2_First_Count_l2"=w390:i32)  [unwired: 11 in]
      n372 = call "BRig_dataLC_Cue2_PostR_OnOff_l2.vi"() -> ("output_Cue2_PostR_OnOff_l2"=w389:i32)  [unwired: 11 in]
      n373 = call "BRig_dataLC_Cue2_PostR_Block_l2.vi"() -> ("output_Cue2_PostR_Block_l2"=w388:i32)  [unwired: 11 in]
      n374 = call "BRig_dataLC_Cue2_PostR_Prob_l2.vi"() -> ("output_Cue2_PostR_Prob_l2"=w387:i32)  [unwired: 11 in]
      n375 = call "BRig_dataLC_Cue2_PostR_Delay_l2.vi"() -> ("output_Cue2_PostR_Delay_l2"=w386:i32)  [unwired: 11 in]
      n376 = call "BRig_dataLC_Cue2_PostR_DelayOpt_l2.vi"() -> ("output_Cue2_PostR_DelayOpt_l2"=w385:i32)  [unwired: 11 in]
      n377 = call "BRig_dataLC_Cue2_PostR_Count_l2.vi"() -> ("output_Cue2_PostR_Count_l2"=w384:i32)  [unwired: 11 in]
      n378 = call "BRig_dataLC_Cue2_PreR_OnOff_l2.vi"() -> ("output_Cue2_PreR_OnOff_l2"=w383:i32)  [unwired: 11 in]
      n379 = call "BRig_dataLC_Cue2_PreR_Block_l2.vi"() -> ("output_Cue2_PreR_Block_l2"=w382:i32)  [unwired: 11 in]
      n380 = call "BRig_dataLC_Cue2_PreR_Prob_l2.vi"() -> ("output_Cue2_PreR_Prob_l2"=w381:i32)  [unwired: 11 in]
      n381 = call "BRig_dataLC_Cue2_PreR_Delay_l2.vi"() -> ("output_Cue2_PreR_Delay_l2"=w380:i32)  [unwired: 11 in]
      n382 = call "BRig_dataLC_Cue2_PreR_DelayOpt_l2.vi"() -> ("output_Cue2_PreR_DelayOpt_l2"=w379:i32)  [unwired: 11 in]
      n383 = call "BRig_dataLC_Cue2_PreR_Count_l2.vi"() -> ("output_Cue2_PreR_Count_l2"=w378:i32)  [unwired: 11 in]
      n384 = local write "LED_baseline"(w545) -> ()
      n385 = local write "Laser_Freq"(w544) -> ()
      n386 = local write "Laser_T"(w543) -> ()
      n387 = local write "Laser_Tpeak"(w542) -> ()
      n388 = local write "Laser_Tshutter"(w541) -> ()
      n389 = local write "Laser_power_min"(w536) -> ()
      n390 = local write "Laser_power_max"(w535) -> ()
      n391 = local write "Laser_power_step"(w534) -> ()
      n392 = Index Array(array=w377, index #1=w395, index #2=w394, index #3=w393, index #4=w392, index #5=w391, index #6=w390, index #7=w389, index #8=w388, index #9=w387, index #10=w386, index #11=w385, index #12=w384, index #13=w383, index #14=w382, index #15=w381, index #16=w380, index #17=w379, index #18=w378) -> (element #1=w501:u16, element #2=w497:u16, element #3=w496:u16, element #4=w495:u16, element #5=w502:u16, element #6=w498:u16, element #7=w503:u16, element #8=w492:u16, element #9=w491:u16, element #10=w490:u16, element #11=w504:u16, element #12=w489:u16, element #13=w505:u16, element #14=w486:u16, element #15=w485:u16, element #16=w484:u16, element #17=w506:u16, element #18=w483:u16)
      n393 = call "BRig_dataLC_Selection_First_OnOff_l2.vi"() -> ("output_Selection_First_OnOff_l2"=w446:i32)  [unwired: 11 in]
      n394 = call "BRig_dataLC_Selection_First_Block_l2.vi"() -> ("output_Selection_First_Block_l2"=w445:i32)  [unwired: 11 in]
      n395 = call "BRig_dataLC_Selection_First_Prob_l2.vi"() -> ("output_Selection_First_Prob_l2"=w444:i32)  [unwired: 11 in]
      n396 = call "BRig_dataLC_Selection_First_Delay_l2.vi"() -> ("output_Selection_First_Delay_l2"=w443:i32)  [unwired: 11 in]
      n397 = call "BRig_dataLC_Selection_First_Count_l2.vi"() -> ("output_Selection_First_Count_l2"=w442:i32)  [unwired: 11 in]
      n398 = call "BRig_dataLC_Selection_PreR_OnOff_l2.vi"() -> ("output_Selection_PreR_OnOff_l2"=w441:i32)  [unwired: 11 in]
      n399 = call "BRig_dataLC_Selection_PreR_Block_l2.vi"() -> ("output_Selection_PreR_Block_l2"=w440:i32)  [unwired: 11 in]
      n400 = call "BRig_dataLC_Selection_PreR_Prob_l2.vi"() -> ("output_Selection_PreR_Prob_l2"=w439:i32)  [unwired: 11 in]
      n401 = call "BRig_dataLC_Selection_PreR_Delay_l2.vi"() -> ("output_Selection_PreR_Delay_l2"=w438:i32)  [unwired: 11 in]
      n402 = call "BRig_dataLC_Selection_PreR_Count_l2.vi"() -> ("output_Selection_PreR_Count_l2"=w437:i32)  [unwired: 11 in]
      n403 = call "BRig_dataLC_Selection_PostR_OnOff_l2.vi"() -> ("output_Selection_PostR_OnOff_l2"=w436:i32)  [unwired: 11 in]
      n404 = call "BRig_dataLC_Selection_PostR_Block_l2.vi"() -> ("output_Selection_PostR_Block_l2"=w435:i32)  [unwired: 11 in]
      n405 = call "BRig_dataLC_Selection_PostR_Prob_l2.vi"() -> ("output_Selection_PostR_Prob_l2"=w434:i32)  [unwired: 11 in]
      n406 = call "BRig_dataLC_Selection_PostR_Delay_l2.vi"() -> ("output_Selection_PostR_Delay_l2"=w433:i32)  [unwired: 11 in]
      n407 = call "BRig_dataLC_Selection_PostR_Count_l2.vi"() -> ("output_Selection_PostR_Count_l2"=w432:i32)  [unwired: 11 in]
      n408 = call "BRig_dataLC_Reward_OnOff_l2.vi"() -> ("output_Reward_OnOff_l2"=w422:i32)  [unwired: 11 in]
      n409 = call "BRig_dataLC_Reward_Block_l2.vi"() -> ("output_Reward_Block_l2"=w423:i32)  [unwired: 11 in]
      n410 = call "BRig_dataLC_Reward_Trial_l2.vi"() -> ("output_Reward_Trial_l2"=w424:i32)  [unwired: 11 in]
      n411 = call "BRig_dataLC_Reward_Prob_l2.vi"() -> ("output_Reward_Prob_l2"=w425:i32)  [unwired: 11 in]
      n412 = call "BRig_dataLC_Reward_Delay_l2.vi"() -> ("output_Reward_Delay_l2"=w426:i32)  [unwired: 11 in]
      n413 = call "BRig_dataLC_Wrong_OnOff_l2.vi"() -> ("output_Wrong_OnOff_l2"=w427:i32)  [unwired: 11 in]
      n414 = call "BRig_dataLC_Wrong_Block_l2.vi"() -> ("output_Wrong_Block_l2"=w428:i32)  [unwired: 11 in]
      n415 = call "BRig_dataLC_Wrong_Trial_l2.vi"() -> ("output_Wrong_Trial_l2"=w429:i32)  [unwired: 11 in]
      n416 = call "BRig_dataLC_Wrong_Prob_l2.vi"() -> ("output_Wrong_Prob_l2"=w430:i32)  [unwired: 11 in]
      n417 = call "BRig_dataLC_Wrong_Delay_l2.vi"() -> ("output_Wrong_Delay_l2"=w431:i32)  [unwired: 11 in]
      n418 = Not Equal To 0?(x=w501) -> (x != 0?=w500:bool)
      n419 = Not Equal To 0?(x=w502) -> (x != 0?=w499:bool)
      n420 = Not Equal To 0?(x=w503) -> (x != 0?=w493:bool)
      n421 = Not Equal To 0?(x=w504) -> (x != 0?=w494:bool)
      n422 = Not Equal To 0?(x=w505) -> (x != 0?=w488:bool)
      n423 = Not Equal To 0?(x=w506) -> (x != 0?=w487:bool)
      n424 = Index Array(array=w547, index #1=w422, index #2=w423, index #3=w424, index #4=w425, index #5=w426, index #6=w427, index #7=w428, index #8=w429, index #9=w430, index #10=w431) -> (element #1=w557:u16, element #2=w556:u16, element #3=w555:u16, element #4=w554:u16, element #5=w553:u16, element #6=w552:u16, element #7=w551:u16, element #8=w550:u16, element #9=w549:u16, element #10=w548:u16)
      n425 = local write "LC_Cue2_First_OnOff"(w500) -> ()
      n426 = local write "LC_Cue2_First_Block"(w497) -> ()
      n427 = local write "LC_Cue2_First_Probability"(w496) -> ()
      n428 = local write "LC_Cue2_First_Tdelay"(w495) -> ()
      n429 = local write "LC_Cue2_First_delayOpt"(w499) -> ()
      n430 = local write "LC_Cue2_First_Count"(w498) -> ()
      n431 = local write "LC_Cue2_PreR_OnOff"(w493) -> ()
      n432 = local write "LC_Cue2_PreR_Block"(w492) -> ()
      n433 = local write "LC_Cue2_PreR_Probability"(w491) -> ()
      n434 = local write "LC_Cue2_PreR_Tdelay"(w490) -> ()
      n435 = local write "LC_Cue2_PreR_delayOpt"(w494) -> ()
      n436 = local write "LC_Cue2_PreR_Count"(w489) -> ()
      n437 = local write "LC_Cue2_PostR_OnOff"(w488) -> ()
      n438 = local write "LC_Cue2_PostR_Block"(w486) -> ()
      n439 = local write "LC_Cue2_PostR_Probability"(w485) -> ()
      n440 = local write "LC_Cue2_PostR_Tdelay"(w484) -> ()
      n441 = local write "LC_Cue2_PostR_delayOpt"(w487) -> ()
      n442 = local write "LC_Cue2_PostR_Count"(w483) -> ()
      n443 = Index Array(array=w547, index #1=w446, index #2=w445, index #3=w444, index #4=w443, index #5=w442, index #6=w441, index #7=w440, index #8=w439, index #9=w438, index #10=w437, index #11=w436, index #12=w435, index #13=w434, index #14=w433, index #15=w432) -> (element #1=w574:u16, element #2=w573:u16, element #3=w572:u16, element #4=w571:u16, element #5=w570:u16, element #6=w569:u16, element #7=w568:u16, element #8=w567:u16, element #9=w566:u16, element #10=w565:u16, element #11=w564:u16, element #12=w563:u16, element #13=w562:u16, element #14=w561:u16, element #15=w560:u16)
      n444 = Not Equal To 0?(x=w557) -> (x != 0?=w559:bool)
      n445 = Not Equal To 0?(x=w552) -> (x != 0?=w558:bool)
      n446 = Not Equal To 0?(x=w574) -> (x != 0?=w577:bool)
      n447 = Not Equal To 0?(x=w569) -> (x != 0?=w576:bool)
      n448 = Not Equal To 0?(x=w564) -> (x != 0?=w575:bool)
      n449 = local write "LC_Reward_OnOff"(w559) -> ()
      n450 = local write "LC_Reward_Block"(w556) -> ()
      n451 = local write "LC_Reward_Trial"(w555) -> ()
      n452 = local write "LC_Reward_Probability"(w554) -> ()
      n453 = local write "LC_Reward_Tdelay"(w553) -> ()
      n454 = local write "LC_Wrong_OnOff"(w558) -> ()
      n455 = local write "LC_Wrong_Block"(w551) -> ()
      n456 = local write "LC_Wrong_Trial"(w550) -> ()
      n457 = local write "LC_Wrong_Probability"(w549) -> ()
      n458 = local write "LC_Wrong_Tdelay"(w548) -> ()
      n459 = local write "LC_Sel_First_OnOff"(w577) -> ()
      n460 = local write "LC_Sel_First_Block"(w573) -> ()
      n461 = local write "LC_Sel_First_Probability"(w572) -> ()
      n462 = local write "LC_Sel_First_Tdelay"(w571) -> ()
      n463 = local write "LC_Sel_First_Count"(w570) -> ()
      n464 = local write "LC_Sel_PreR_OnOff"(w576) -> ()
      n465 = local write "LC_Sel_PreR_Block"(w568) -> ()
      n466 = local write "LC_Sel_PreR_Probability"(w567) -> ()
      n467 = local write "LC_Sel_PreR_Tdelay"(w566) -> ()
      n468 = local write "LC_Sel_PreR_Count"(w565) -> ()
      n469 = local write "LC_Sel_PostR_OnOff"(w575) -> ()
      n470 = local write "LC_Sel_PostR_Block"(w563) -> ()
      n471 = local write "LC_Sel_PostR_Probability"(w562) -> ()
      n472 = local write "LC_Sel_PostR_Tdelay"(w561) -> ()
      n473 = local write "LC_Sel_PostR_Count"(w560) -> ()
    }
  }
  "output_dataLC" <- w4
  "output_dataExp" <- w1
